vi "Go.vi"(9 "Timing Data":T1(array[cluster]), 10 "Control In":T2={"I-O.lvclass"=refnum, "Gantry"=refnum, "Dispenser"="COM1"}, 11 "Sensor Dispense in":refnum<class "Sensor Dispense.lvclass">) -> (2 "Control Out":T2={"I-O.lvclass"=refnum, "Gantry"=refnum, "Dispenser"="COM1"}, 3 "Sensor Dispense out":refnum<class "Sensor Dispense.lvclass">)   [LabVIEW 2021, in "Sensor Dispense.lvclass"]
uses:
  Sensor Dispense.lvclass
  C:/Users/HEP/Documents/GitHub/Gantry/UCSB-Gantry-HEP-main/Classes/Routine/Dispense/Dispense.lvclass
  Classes/Controller/Controllers.ctl
  Classes/Controller/I-O/I-O.lvclass
  C:/Program Files (x86)/Aerotech/A3200/LabVIEW/2010/Bin/Aerotech.A3200.dll
  Program Files (x86)/Aerotech/A3200/LabVIEW/2010/Bin/Aerotech.A3200.dll
  Sensor Dispense.lvclass/Sensor Dispense.ctl
  Classes/Controller/Motion/Motion.lvclass
  Classes/Controller/Dispenser/Dispenser.lvclass
  Classes/Controller/Motion/A3200/A3200.lvclass
  Classes/Controller/Controller.lvclass
panel:
  out "error out":errorcluster
  in  "error in (no error)":errorcluster
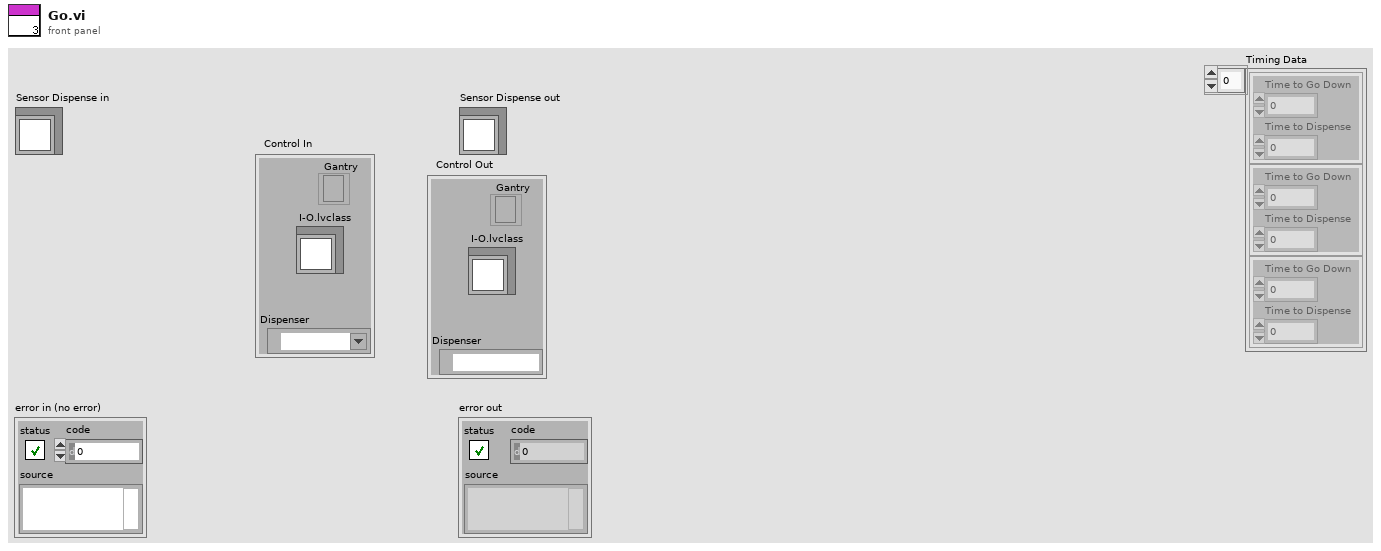
[diagram p1: front panel]
types:
  T1 = cluster{"Time to Go Down":i32, "Time to Dispense":i32}[]
  T2 = typedef "Controller.lvclass/Controllers.ctl" = cluster{"I-O.lvclass":refnum<class "I-O.lvclass">, "Gantry":refnum<k24>, "Dispenser":refnum<visa-resource-name>}
  T3 = cluster{"Endpoints":dbl[][], "Center":dbl[], "CW/CCW":dbl, "Dispense Type":enum16{"N-gon", "Square", "Arc", "Dot", "Line", "Circle"}}[]
  T4 = cluster{"Endpoints":dbl[][], "Center":dbl[], "CW/CCW":dbl, "Dispense Type":enum16{"N-gon", "Square", "Arc", "Dot", "Line", "Circle"}}
  T5 = enum16{"N-gon", "Square", "Arc", "Dot", "Line", "Circle"}
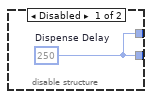
[diagram p2: hidden frame]
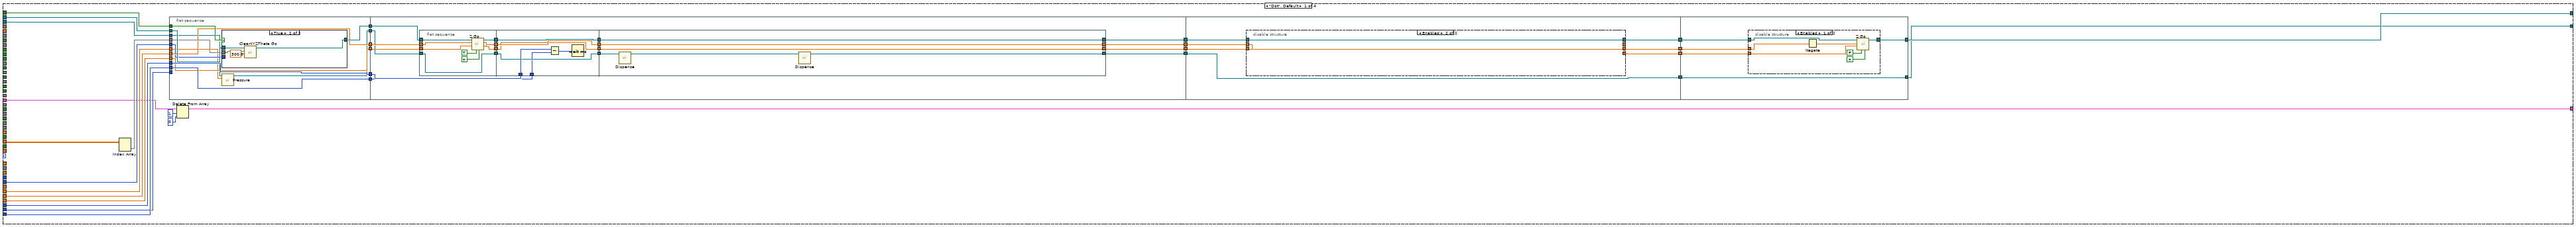
[diagram p4: hidden frame]
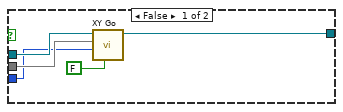
[diagram p5: hidden frame]
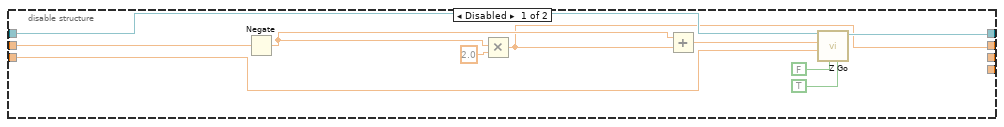
[diagram p6: hidden frame]
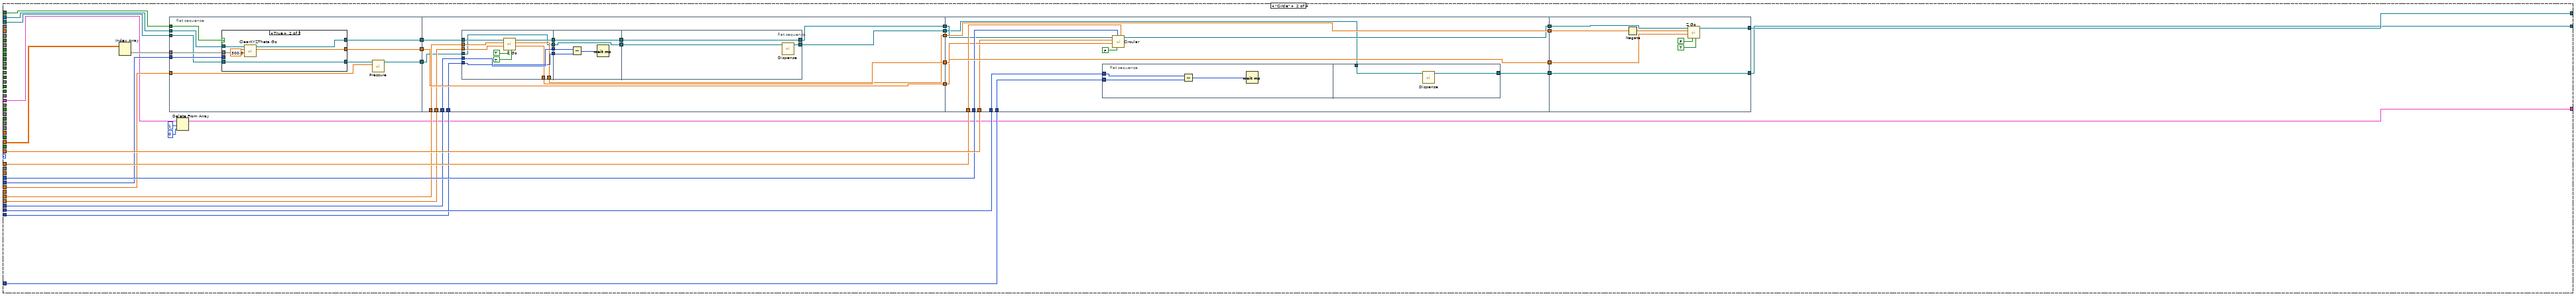
[diagram p8: hidden frame]
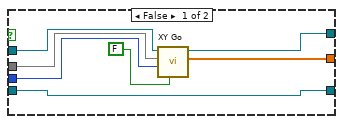
[diagram p9: hidden frame]
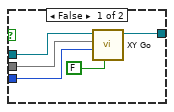
[diagram p10: hidden frame]
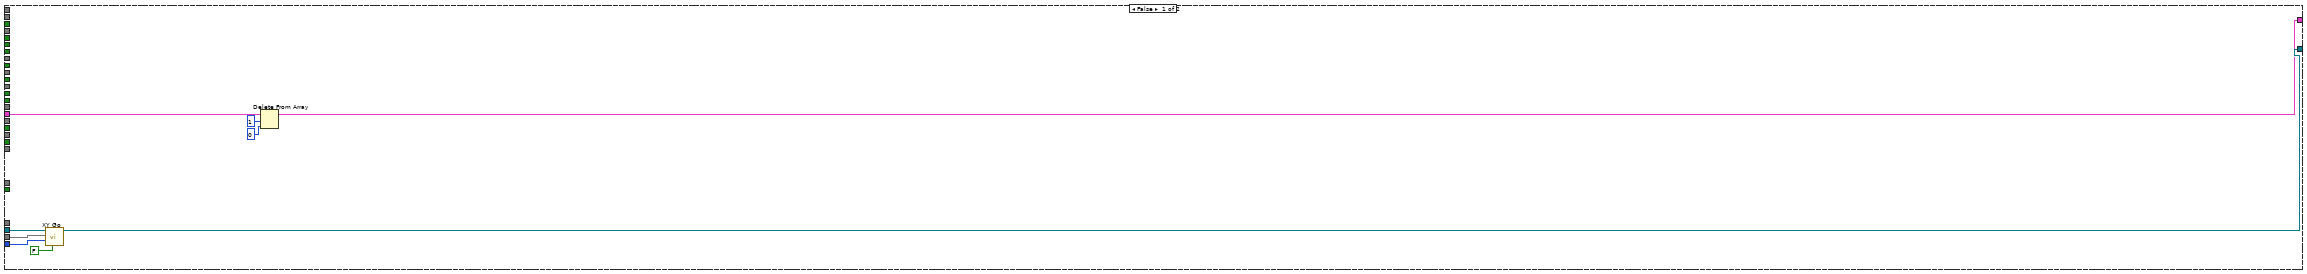
[diagram p11: hidden frame]
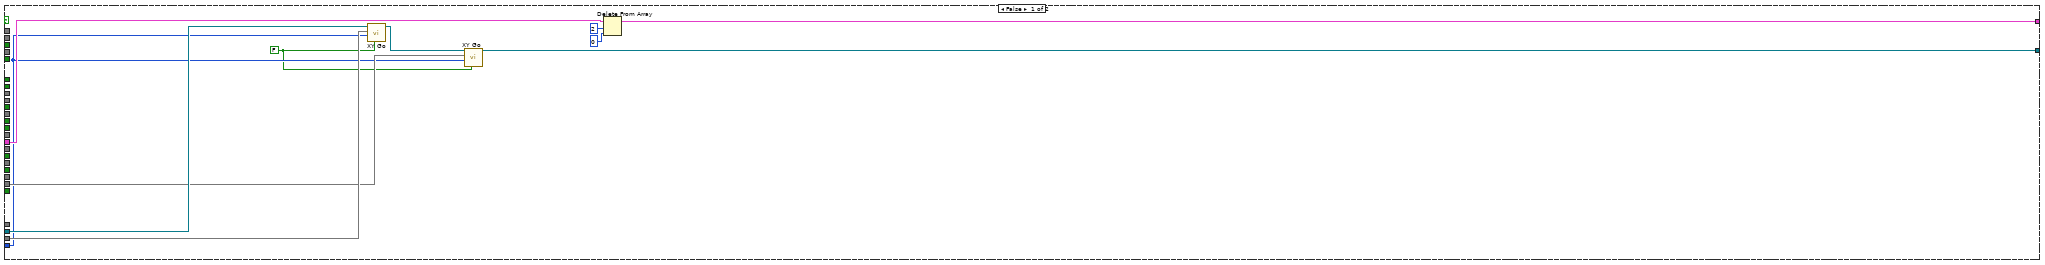
[diagram p12: hidden frame]
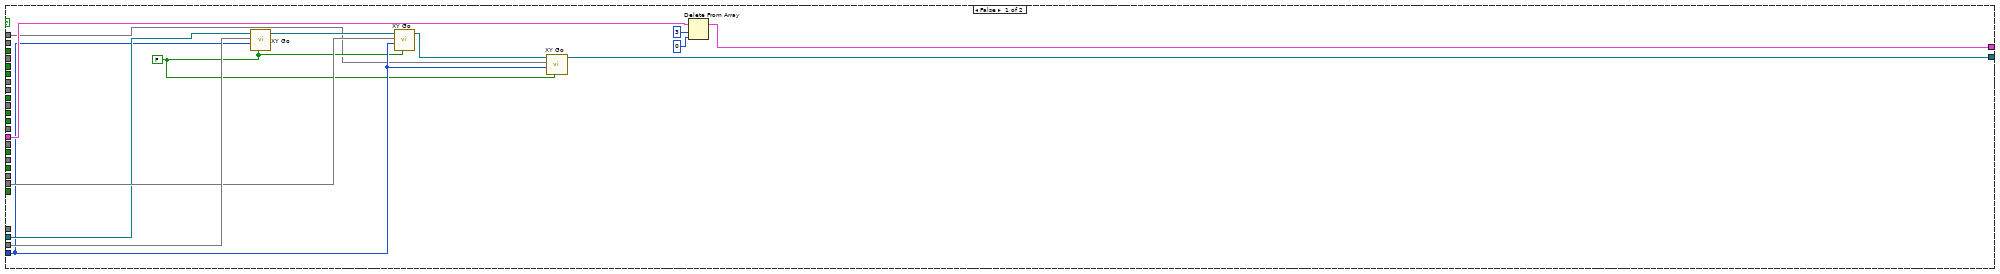
[diagram p13: hidden frame]
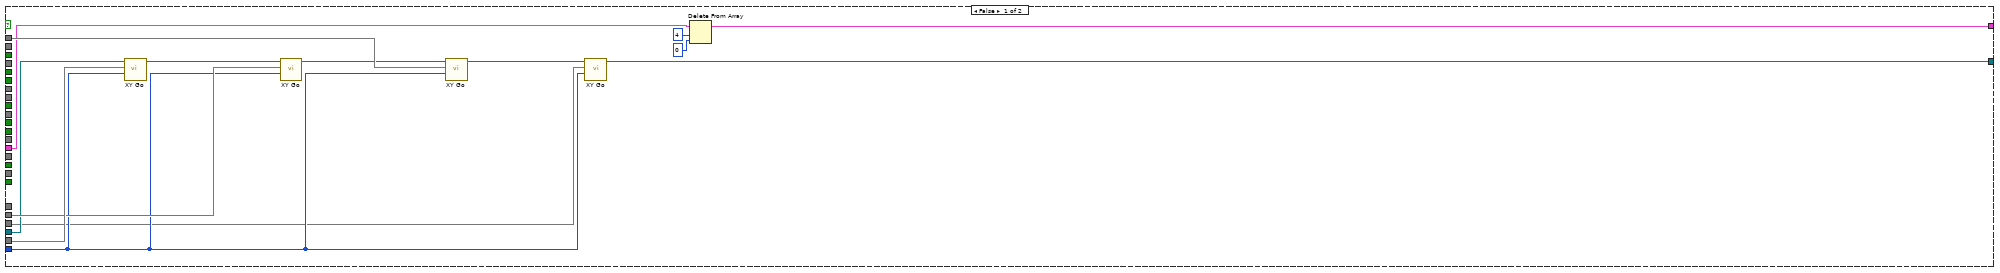
[diagram p14: hidden frame]
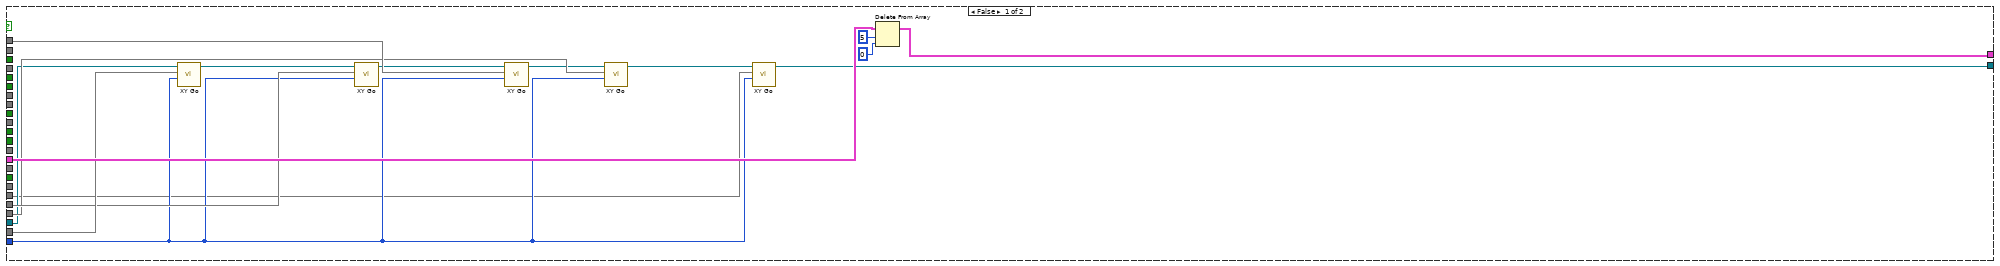
[diagram p15: hidden frame]
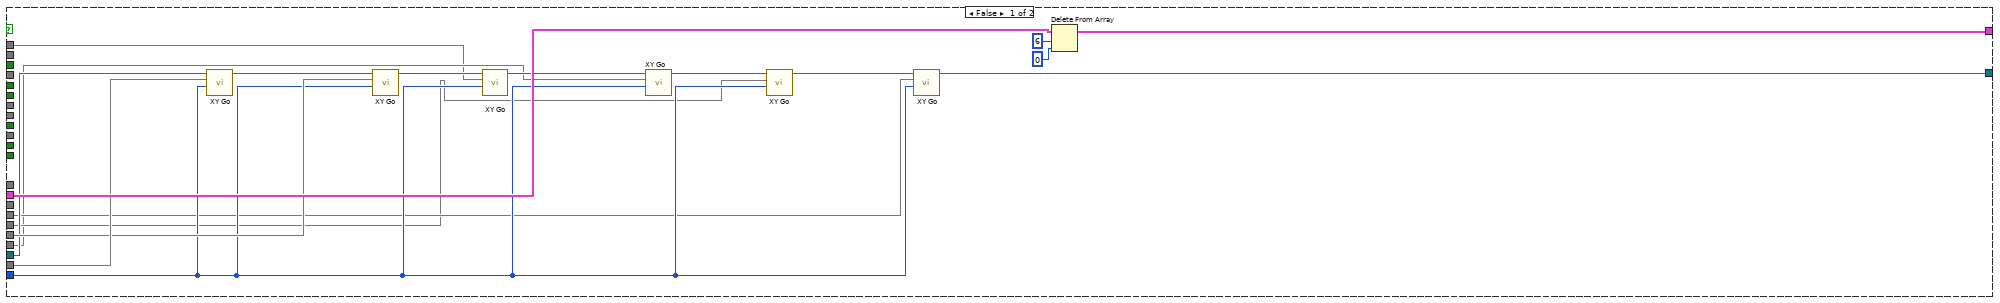
[diagram p16: hidden frame]
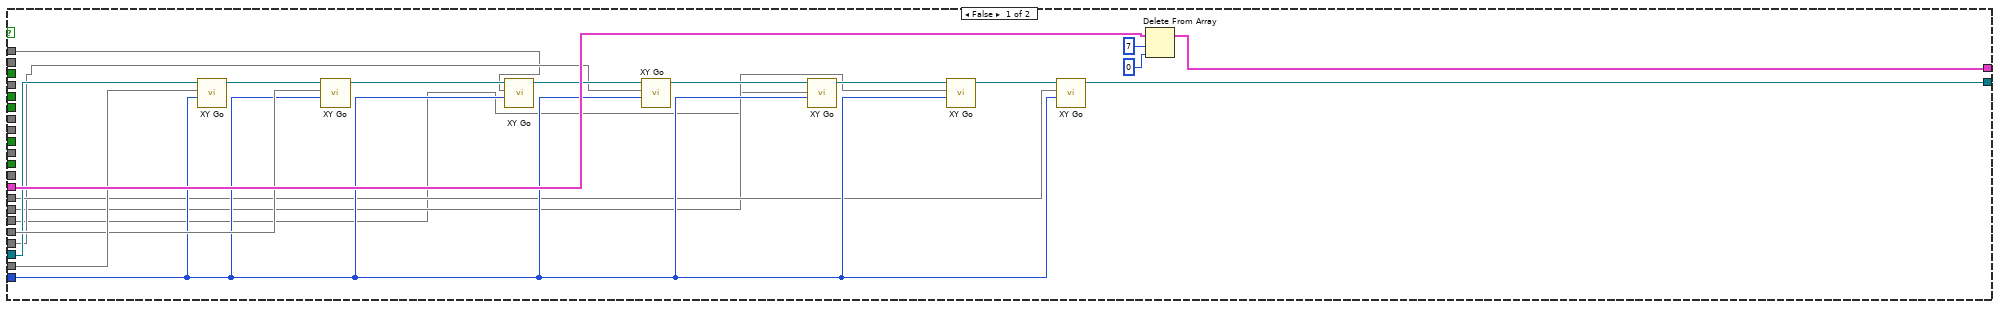
[diagram p17: hidden frame]
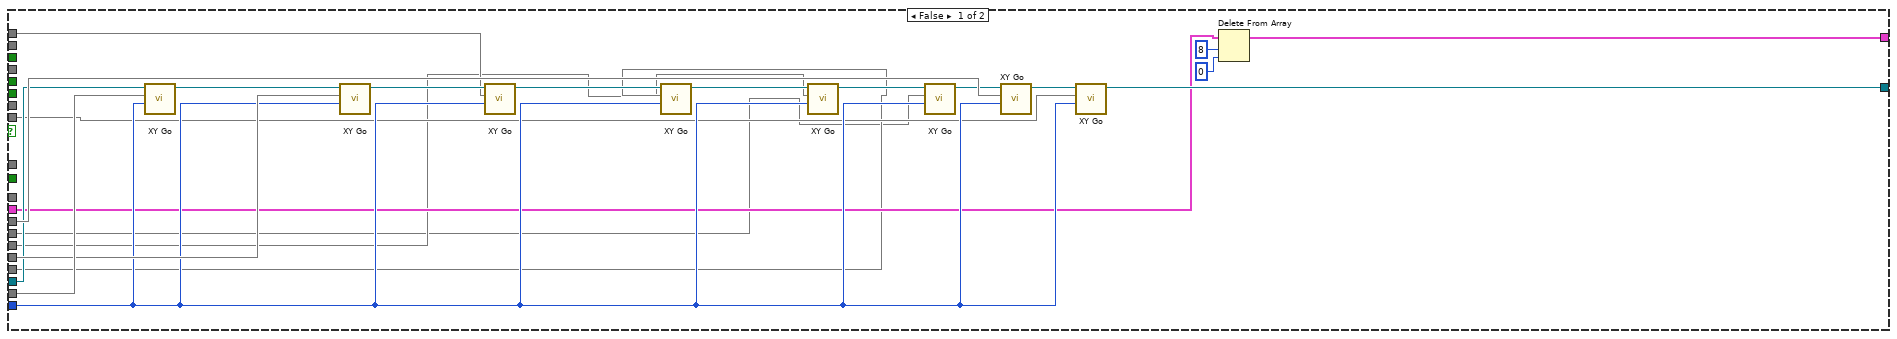
[diagram p18: hidden frame]
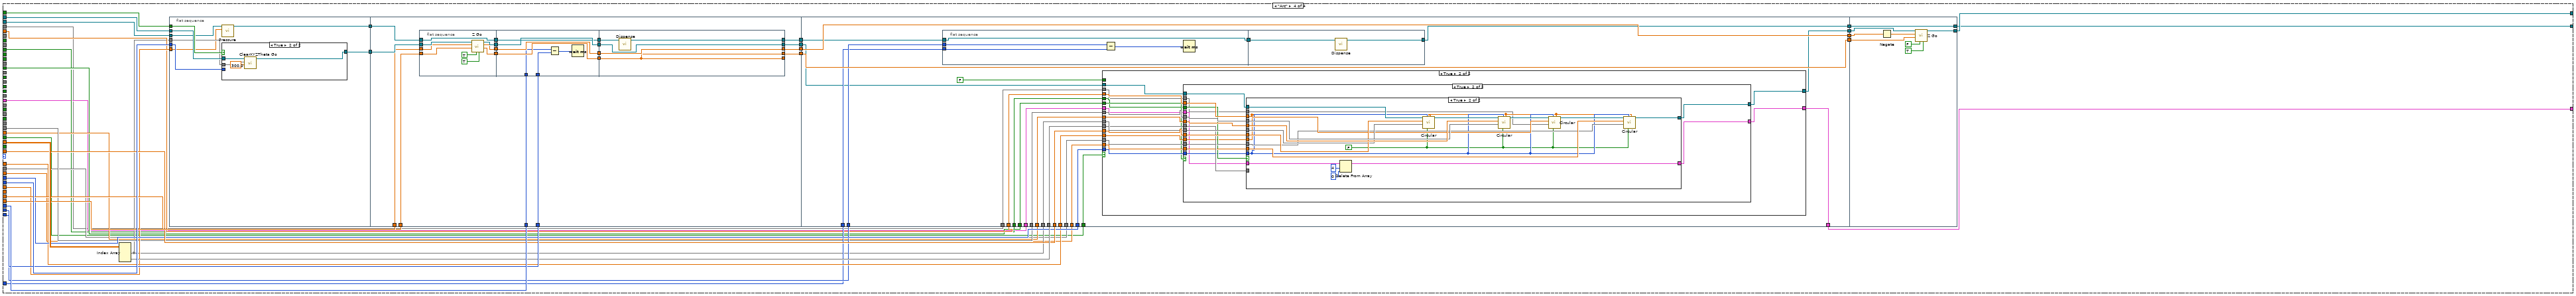
[diagram p19: hidden frame]
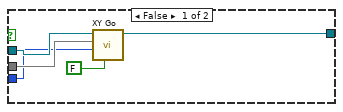
[diagram p20: hidden frame]
diagram:
  n1 = case shown="No Error" "error in (no error)" {
    selector: "error in (no error)" -> [w7 w1398]
    tunnel: "Sensor Dispense in" -> [w12 w1397]
    tunnel: [w11 w1397] -> w5
    tunnel: "Control In" -> [w10 w1396]
    tunnel: [w9 w1396] -> w3
    tunnel: [w8 w1398] -> w2
    frame No Error {
      n2 = in-place {
        in-place-border: w12 -> [w24]
        in-place-border: [w23] -> w11
        in-place-border: w7 -> [w17]
        in-place-border: [w16] -> w8
        n3 = in-place-cluster #1(w10) -> ("Gantry"=w25:refnum<k24>, "Dispenser"=w20:refnum<visa-resource-name>)
        n4 = Unbundle By Name(w24) -> ("Dispense Steps"=w21:T3, "Glue Speed"=w15:i32, "Move Speed"=w26:i32, "Line Pressure"=w13:dbl, "Dot Pressure"=w14:dbl)
        n5 = while {
          tunnel: w26 -> [w170]
          shift-right: [w163] -> w22
          shift-left: w25 -> [w31]
          tunnel: w15 -> [w169]
          shift-right: [w155] -> w23
          shift-left: w24 -> [w167]
          shift-right: [w158] -> w18
          shift-left: w20 -> [w161]
          tunnel: "Timing Data" -> [w160] mode=indexing
          shift-right: [w29] -> w16
          shift-left: w17 -> [w28]
          tunnel: w14 -> [w153]
          tunnel: w13 -> [w152]
          shift-right: [w116] -> _
          shift-left: w21 -> [w68]
          i -> [w166]
          stop <- w118 stop-if-true
          # "740 is good"
          # "compares 3 and 4"
          # "compares 2 and 3"
          # "Compares 1 and 2"
          # "#2"
          # "#3"
          # "#4"
          # "#3"
          # "1/11/23 - Originally 750"
          n6 = Unbundle By Name(w160) -> ("Time to Go Down"=w159:i32, "Time to Dispense"=w150:i32)
          n7 = call "get Estop status.vi"("error in (no error)"=w28, "controller in"=w31) -> ("error out"=w29:errorcluster, "Estop?"=w27:bool, "controller out"=w30:refnum<k24>)  [unwired: 7 in]
          n8 = disable-structure shown="Enabled" {
            disable-tunnel: [w171 w175] -> w154
            disable-tunnel: [w171 w173] -> w151
            disable-tunnel: w150 -> [_ w174]
            frame Disabled {
              w171 = 250  # Dispense Delay
            }
            frame Enabled {
              w172 = 450  # End Dispense Delay
              w175 = 740  # Start Dispense Delay
              # "For arcs it is set to 250"
              # "525 - 1/23/2023"
              # "Originally 0"
              n9 = disable-structure shown="Disabled" {
                disable-tunnel: w174 -> [w180 _]
                disable-tunnel: [w177 w181] -> w173
                disable-tunnel: w172 -> [w176 w181]
                frame Disabled {
                  n10 = Less?(x=w180, y=w176) -> (x < y?=w179:bool)
                  n11 = Select(t=0, s=w179, f=w176) -> (s? t:f=w177:i32)
                }
                frame Enabled {
                }
              }
            }
          }
          n12 = Stop(stop? (T)=w27) -> ()
          n13 = Index Array(array=w68) -> (element=w148:T4)  [unwired: 1 in]
          n14 = Index Array(array=w68, index=11) -> (element=w74:T4)
          n15 = Index Array(array=w68, index=7) -> (element=w109:T4)
          n16 = Index Array(array=w68, index=9) -> (element=w80:T4)
          n17 = Index Array(array=w68, index=10) -> (element=w77:T4)
          n18 = Index Array(array=w68, index=12) -> (element=w71:T4)
          n19 = Index Array(array=w68, index=2) -> (element=w145:T4)
          n20 = Index Array(array=w68, index=8) -> (element=w83:T4)
          n21 = Index Array(array=w68, index=4) -> (element=w115:T4)
          n22 = Index Array(array=w68, index=6) -> (element=w111:T4)
          n23 = Index Array(array=w68, index=5) -> (element=w113:T4)
          n24 = Index Array(array=w68, index=1) -> (element=w147:T4)
          n25 = Index Array(array=w68, index=3) -> (element=w144:T4)
          n26 = Unbundle By Name(w145) -> ("Endpoints"=w142:dbl[][], "Center"=w123:dbl[])
          n27 = Unbundle By Name(w80) -> ("Endpoints"=w79:dbl[][])  [unwired: 1 out]
          n28 = Unbundle By Name(w109) -> ("Endpoints"=w108:dbl[][])  [unwired: 1 out]
          n29 = Unbundle By Name(w83) -> ("Endpoints"=w82:dbl[][])  [unwired: 1 out]
          n30 = Unbundle By Name(w115) -> ("Endpoints"=w114:dbl[][])  [unwired: 1 out]
          n31 = Unbundle By Name(w148) -> ("Endpoints"=w139:dbl[][], "Center"=w162:dbl[], "Dispense Type"=w164:T5, "CW/CCW"=w168:dbl)
          n32 = Unbundle By Name(w111) -> ("Endpoints"=w110:dbl[][])  [unwired: 1 out]
          n33 = Unbundle By Name(w144) -> ("Endpoints"=w143:dbl[][], "Center"=w122:dbl[])
          n34 = Unbundle By Name(w113) -> ("Endpoints"=w112:dbl[][])  [unwired: 1 out]
          n35 = Unbundle By Name(w147) -> ("Endpoints"=w146:dbl[][], "Center"=w124:dbl[])
          n36 = Unbundle By Name(w74) -> ("Endpoints"=w73:dbl[][])  [unwired: 1 out]
          n37 = Unbundle By Name(w77) -> ("Endpoints"=w76:dbl[][])  [unwired: 1 out]
          n38 = Unbundle By Name(w71) -> ("Endpoints"=w70:dbl[][])  [unwired: 1 out]
          n39 = Index Array(array=w108) -> (element #1=w87:dbl[], element #2=w66:dbl[])  [unwired: 4 in]
          n40 = Index Array(array=w142) -> (element #1=w136:dbl[], element #2=w32:dbl[])  [unwired: 4 in]
          n41 = Index Array(array=w112) -> (element #1=w98:dbl[], element #2=w36:dbl[])  [unwired: 4 in]
          n42 = Index Array(array=w143) -> (element #1=w135:dbl[], element #2=w33:dbl[])  [unwired: 4 in]
          n43 = Index Array(array=w82) -> (element #1=w67:dbl[], element #2=w60:dbl[])  [unwired: 4 in]
          n44 = Index Array(array=w79) -> (element #1=w61:dbl[], element #2=w54:dbl[])  [unwired: 4 in]
          n45 = Index Array(array=w114) -> (element #1=w103:dbl[], element #2=w35:dbl[])  [unwired: 4 in]
          n46 = Index Array(array=w110) -> (element #1=w93:dbl[], element #2=w34:dbl[])  [unwired: 4 in]
          n47 = Index Array(array=w146) -> (element #1=w137:dbl[], element #2=w125:dbl[])  [unwired: 4 in]
          n48 = Index Array(array=w73) -> (element #1=w48:dbl[], element #2=w43:dbl[])  [unwired: 4 in]
          n49 = Index Array(array=w76) -> (element #1=w55:dbl[], element #2=w49:dbl[])  [unwired: 4 in]
          n50 = Index Array(array=w70) -> (element #1=w42:dbl[], element #2=w37:dbl[])  [unwired: 4 in]
          n51 = Index Array(array=w139) -> (element #2=w138:dbl[])  [unwired: 4 in, 1 out]
          n52 = Equal?(x=w43, y=w42) -> (x = y?=w41:bool[])
          n53 = Equal?(x=w49, y=w48) -> (x = y?=w47:bool[])
          n54 = Equal?(x=w54, y=w55) -> (x = y?=w53:bool[])
          n55 = Equal?(x=w125, y=w136) -> (x = y?=w131:bool[])
          n56 = Equal?(x=w66, y=w67) -> (x = y?=w65:bool[])
          n57 = Equal?(x=w60, y=w61) -> (x = y?=w59:bool[])
          n58 = Equal?(x=w34, y=w87) -> (x = y?=w88:bool[])
          n59 = Equal?(x=w36, y=w93) -> (x = y?=w92:bool[])
          n60 = Equal?(x=w35, y=w98) -> (x = y?=w97:bool[])
          n61 = Equal?(x=w33, y=w103) -> (x = y?=w102:bool[])
          n62 = Equal?(x=w32, y=w135) -> (x = y?=w130:bool[])
          n63 = Index Array(array=w130) -> (element #1=w127:bool, element #2=w126:bool)  [unwired: 2 in]
          n64 = And(x=w127, y=w126) -> (x .and. y?=w119:bool)
          n65 = Index Array(array=w41) -> (element #1=w40:bool, element #2=w39:bool)  [unwired: 2 in]
          n66 = Equal?(x=w138, y=w137) -> (x = y?=w134:bool[])
          n67 = Index Array(array=w53) -> (element #1=w52:bool, element #2=w51:bool)  [unwired: 2 in]
          n68 = Index Array(array=w131) -> (element #1=w129:bool, element #2=w128:bool)  [unwired: 2 in]
          n69 = Index Array(array=w65) -> (element #1=w64:bool, element #2=w63:bool)  [unwired: 2 in]
          n70 = Index Array(array=w59) -> (element #1=w58:bool, element #2=w57:bool)  [unwired: 2 in]
          n71 = Index Array(array=w88) -> (element #1=w86:bool, element #2=w85:bool)  [unwired: 2 in]
          n72 = Index Array(array=w92) -> (element #1=w91:bool, element #2=w90:bool)  [unwired: 2 in]
          n73 = Index Array(array=w97) -> (element #1=w96:bool, element #2=w95:bool)  [unwired: 2 in]
          n74 = property on="Property Node" class="Sensor Dispense.lvclass"(reference=w167) -> (reference out=w155:refnum<class "Sensor Dispense.lvclass">, "Z height"=w157:dbl, "Z speed"=w156:dbl)  [unwired: 1 in, 1 out]
          n75 = Index Array(array=w47) -> (element #1=w46:bool, element #2=w45:bool)  [unwired: 2 in]
          n76 = Index Array(array=w102) -> (element #1=w101:bool, element #2=w100:bool)  [unwired: 2 in]
          n77 = And(x=w40, y=w39) -> (x .and. y?=w38:bool)
          n78 = Index Array(array=w134) -> (element #1=w133:bool, element #2=w132:bool)  [unwired: 2 in]
          n79 = And(x=w46, y=w45) -> (x .and. y?=w44:bool)
          n80 = And(x=w52, y=w51) -> (x .and. y?=w50:bool)
          n81 = And(x=w64, y=w63) -> (x .and. y?=w62:bool)
          n82 = And(x=w58, y=w57) -> (x .and. y?=w56:bool)
          n83 = And(x=w86, y=w85) -> (x .and. y?=w84:bool)
          n84 = And(x=w91, y=w90) -> (x .and. y?=w89:bool)
          n85 = And(x=w96, y=w95) -> (x .and. y?=w94:bool)
          n86 = And(x=w101, y=w100) -> (x .and. y?=w99:bool)
          n87 = And(x=w129, y=w128) -> (x .and. y?=w120:bool)
          n88 = And(x=w133, y=w132) -> (x .and. y?=w121:bool)
          n89 = Equal To 0?(x=w166) -> (x = 0?=w165:bool)
          n90 = case shown="\"Line\"" w164 {
            tunnel: w162 -> [_ w337 _ w1187]
            tunnel: w30 -> [w212 w338 w489 w1195]
            tunnel: w170 -> [w195 w331 w488 w1193]
            tunnel: [w211 w341 w485 w1183] -> w163
            tunnel: w169 -> [_ w336 w476 w1186]
            tunnel: w168 -> [_ w335 _ w1185]
            tunnel: w156 -> [w203 w333 w473 w1189]
            tunnel: w157 -> [w204 w334 w474 w1190]
            tunnel: w165 -> [w213 w332 w487 w1196]
            tunnel: w161 -> [w202 w315 w480 w1179]
            tunnel: w159 -> [w200 w322 w478 w1192]
            tunnel: w150 -> [w205 w323 w475 w1184]
            tunnel: w154 -> [w206 w321 w479 w1191]
            tunnel: [w210 w316 w483 w1182] -> w158
            tunnel: w139 -> [w209 w320 w482 w1194]
            tunnel: w153 -> [w194 _ _ _]
            tunnel: w152 -> [_ w313 w456 w1178]
            tunnel: w151 -> [_ w312 w455 w1177]
            tunnel: w125 -> [_ _ w452 w1176]
            tunnel: w124 -> [_ _ _ w1175]
            tunnel: w123 -> [_ _ _ w1174]
            tunnel: w122 -> [_ _ _ w1172]
            tunnel: w33 -> [_ _ w447 w1171]
            tunnel: w121 -> [_ _ w450 w1170]
            tunnel: w120 -> [_ _ w449 w1169]
            tunnel: w119 -> [_ _ w448 w1168]
            tunnel: w68 -> [w186 w311 w453 w1167]
            tunnel: [w183 w308 w454 w1166] -> w116
            tunnel: w32 -> [_ _ w451 w1165]
            tunnel: w99 -> [_ _ w446 _]
            tunnel: w35 -> [_ _ w445 _]
            tunnel: w94 -> [_ _ w444 _]
            tunnel: w36 -> [_ _ w443 _]
            tunnel: w89 -> [_ _ w442 _]
            tunnel: w84 -> [_ _ w441 _]
            tunnel: w34 -> [_ _ w440 _]
            tunnel: w66 -> [_ _ w439 _]
            tunnel: w62 -> [_ _ w438 _]
            tunnel: w60 -> [_ _ w437 _]
            tunnel: w56 -> [_ _ w436 _]
            tunnel: w54 -> [_ _ w435 _]
            tunnel: w50 -> [_ _ w434 _]
            tunnel: w49 -> [_ _ w433 _]
            tunnel: w44 -> [_ _ w432 _]
            tunnel: w43 -> [_ _ w431 _]
            tunnel: w38 -> [_ _ w430 _]
            tunnel: w37 -> [_ _ w429 _]
            frame "Dot", Default {
              n91 = Index Array(array=w209) -> (element=w208:dbl[])  [unwired: 2 in]
              n92 = flat-sequence {
                tunnel: w213 -> [w225]
                tunnel: w212 -> [w224]
                tunnel: w208 -> [w223]
                tunnel: [w222] -> w207
                tunnel: w206 -> [w219]
                tunnel: w205 -> [_]
                tunnel: w204 -> [w221]
                tunnel: w203 -> [w218]
                tunnel: w202 -> [w216]
                tunnel: [w221] -> w201
                tunnel: w200 -> [w220]
                tunnel: [w220] -> w199
                tunnel: [w219] -> w198
                tunnel: [w215] -> w197
                tunnel: [w218] -> w196
                tunnel: w195 -> [w217]
                tunnel: w194 -> [w214]
                tunnel: [w252] -> w191
                tunnel: w207 -> [w251]
                tunnel: [w248] -> w190
                tunnel: w201 -> [w247]
                tunnel: w199 -> [w246]
                tunnel: w198 -> [w245]
                tunnel: w197 -> [w244]
                tunnel: w196 -> [w241]
                tunnel: [w239] -> w189
                tunnel: [w238] -> w188
                tunnel: w191 -> [w280]
                tunnel: w190 -> [w279]
                tunnel: w189 -> [w278]
                tunnel: w188 -> [w277]
                tunnel: [w281] -> w193
                tunnel: [w280] -> w192
                tunnel: [w275] -> w187
                tunnel: [w276] -> w182
                tunnel: [w295] -> w210
                tunnel: [w298] -> w211
                tunnel: w193 -> [w299]
                tunnel: w192 -> [w295]
                tunnel: w187 -> [w297]
                tunnel: w182 -> [w296]
                frame #0 {
                  n93 = case shown="True" w225 {
                    tunnel: w224 -> [w230 w234]
                    tunnel: [w229 w233] -> w222
                    tunnel: w223 -> [w228 w232]
                    tunnel: w217 -> [w227 _]
                    frame False {
                      n94 = call "XY Go.vi"("return immediately"=FALSE, "Speed"=w227, "XY In"=w228, "Gantry In"=w230) -> ("Gantry Out"=w229:refnum<k24>)  [unwired: 5 in, 2 out]
                    }
                    frame True {
                      n95 = call "ClearXYZTheta Go.vi"("Speed"=300.0, "XYZTheta In"=w232, "Gantry In"=w234) -> ("Gantry Out"=w233:refnum<k24>)  [unwired: 6 in, 2 out]
                    }
                  }
                  n96 = call "Pressure.vi"("Pressure"=w214, "VISA resource name"=w216) -> ("VISA resource name out"=w215:refnum<visa-resource-name>)  [unwired: 8 in, 1 out]
                }
                frame #1 {
                  n97 = flat-sequence {
                    tunnel: w251 -> [w261]
                    tunnel: [w260] -> w249
                    tunnel: w247 -> [w254]
                    tunnel: w244 -> [w258]
                    tunnel: [w258] -> w243
                    tunnel: w241 -> [w257]
                    tunnel: [w256] -> w236
                    tunnel: [w253] -> w235
                    tunnel: [w268] -> w250
                    tunnel: w249 -> [w268]
                    tunnel: w246 -> [w267]
                    tunnel: w245 -> [w263]
                    tunnel: w243 -> [w266]
                    tunnel: [w266] -> w242
                    tunnel: [w265] -> w240
                    tunnel: [w264] -> w237
                    tunnel: w236 -> [w264]
                    tunnel: w235 -> [w265]
                    tunnel: [w274] -> w252
                    tunnel: w250 -> [w273]
                    tunnel: [w273] -> w248
                    tunnel: w242 -> [w272]
                    tunnel: w240 -> [w270]
                    tunnel: [w270] -> w239
                    tunnel: [w269] -> w238
                    tunnel: w237 -> [w269]
                    frame #0 {
                      n98 = call "Z Go.vi"("Increment"=TRUE, "Return Immediately"=TRUE, "Speed In"=w257, "Position In"=w254, "Gantry In"=w261) -> ("Speed Out"=w256:dbl, "Position Out"=w253:dbl, "Gantry Out"=w260:refnum<k24>)  [unwired: 3 in, 1 out]
                    }
                    frame #1 {
                      n99 = Subtract(x=w267, y=w263) -> (x-y=w262:i32)
                      n100 = Wait (ms)(milliseconds to wait=w262) -> ()  [unwired: 1 out]
                    }
                    frame #2 {
                      n101 = call "Dispense.vi"("Dispenser In"=w272) -> ("Dispenser Out"=w271:refnum<visa-resource-name>)  [unwired: 9 in, 1 out]
                      n102 = call "Dispense.vi"("Dispenser In"=w271) -> ("Dispenser Out"=w274:refnum<visa-resource-name>)  [unwired: 9 in, 1 out]
                    }
                  }
                }
                frame #2 {
                  n103 = disable-structure shown="Enabled" {
                    disable-tunnel: [w291 w294] -> w281
                    disable-tunnel: w279 -> [w290 w294]
                    disable-tunnel: w278 -> [w289 w292]
                    disable-tunnel: w277 -> [w286 w293]
                    disable-tunnel: [w282 _] -> _
                    disable-tunnel: [_ w293] -> w276
                    disable-tunnel: [_ w292] -> w275
                    frame Disabled {
                      n104 = Negate(x=w289) -> (-x=w284:dbl)
                      n105 = Multiply(x=w284, y=2.0) -> (x*y=w282:dbl)
                      n106 = Add(x=w284, y=w282) -> (x+y=w285:dbl)
                      n107 = call "Z Go.vi"("Increment"=TRUE, "Return Immediately"=FALSE, "Speed In"=w286, "Position In"=w285, "Gantry In"=w290) -> ("Gantry Out"=w291:refnum<k24>)  [unwired: 3 in, 3 out]
                    }
                    frame Enabled {
                    }
                  }
                }
                frame #3 {
                  n108 = disable-structure shown="Enabled" {
                    disable-tunnel: w299 -> [w306 w307]
                    disable-tunnel: [w305 w307] -> w298
                    disable-tunnel: w297 -> [w300 _]
                    disable-tunnel: w296 -> [w301 _]
                    frame Enabled {
                      n109 = Negate(x=w300) -> (-x=w304:dbl)
                      n110 = call "Z Go.vi"("Increment"=TRUE, "Return Immediately"=FALSE, "Speed In"=w301, "Position In"=w304, "Gantry In"=w306) -> ("Gantry Out"=w305:refnum<k24>)  [unwired: 3 in, 3 out]
                    }
                    frame Disabled {
                    }
                  }
                }
              }
              n111 = Delete From Array(array=w186, length=1, index=0) -> (array with subset deleted=w183:T3)  [unwired: 1 out]
            }
            frame "Circle" {
              n112 = Index Array(array=w320) -> (element=w319:dbl[])  [unwired: 2 in]
              n113 = flat-sequence {
                tunnel: [w349] -> w340
                tunnel: w338 -> [w350]
                tunnel: w332 -> [w351]
                tunnel: w331 -> [w348]
                tunnel: [w347] -> w329
                tunnel: w319 -> [w346]
                tunnel: w315 -> [w345]
                tunnel: [w343] -> w314
                tunnel: w313 -> [w342]
                tunnel: w334 -> [w374]
                tunnel: w333 -> [w375]
                tunnel: [w381] -> w330
                tunnel: [w372] -> w328
                tunnel: [w373] -> w327
                tunnel: w329 -> [w381]
                tunnel: w340 -> [w371]
                tunnel: [w380] -> w324
                tunnel: w322 -> [w379]
                tunnel: w321 -> [w378]
                tunnel: [w368] -> w318
                tunnel: w314 -> [w367]
                tunnel: [w403] -> w339
                tunnel: [w413] -> w326
                tunnel: [w412] -> w325
                tunnel: w323 -> [w411]
                tunnel: w324 -> [w401]
                tunnel: w330 -> [w406]
                tunnel: w328 -> [w413]
                tunnel: w327 -> [w412]
                tunnel: w335 -> [w409]
                tunnel: w336 -> [w407]
                tunnel: w337 -> [w405]
                tunnel: w318 -> [w404]
                tunnel: [w410] -> w317
                tunnel: w312 -> [w402]
                tunnel: [w424] -> w341
                tunnel: w339 -> [w425]
                tunnel: w326 -> [w426]
                tunnel: w325 -> [w423]
                tunnel: w317 -> [w422]
                tunnel: [w422] -> w316
                frame #0 {
                  n114 = case shown="True" w351 {
                    tunnel: w350 -> [w358 w364]
                    tunnel: [w357 w363] -> w349
                    tunnel: w348 -> [w356 _]
                    tunnel: [w355 w361] -> w347
                    tunnel: w346 -> [w354 w362]
                    tunnel: w345 -> [w353 w360]
                    tunnel: [w353 w360] -> w344
                    frame False {
                      n115 = call "XY Go.vi"("return immediately"=FALSE, "Speed"=w356, "XY In"=w354, "Gantry In"=w358) -> ("XY Out"=w355:dbl[], "Gantry Out"=w357:refnum<k24>)  [unwired: 5 in, 1 out]
                    }
                    frame True {
                      n116 = call "ClearXYZTheta Go.vi"("Speed"=300.0, "XYZTheta In"=w362, "Gantry In"=w364) -> ("XYZTheta Out"=w361:dbl[], "Gantry Out"=w363:refnum<k24>)  [unwired: 6 in, 1 out]
                    }
                  }
                  n117 = call "Pressure.vi"("Pressure"=w342, "VISA resource name"=w344) -> ("VISA resource name out"=w343:refnum<visa-resource-name>)  [unwired: 8 in, 1 out]
                }
                frame #1 {
                  n118 = flat-sequence {
                    tunnel: w378 -> [w391]
                    tunnel: w379 -> [w392]
                    tunnel: [w392] -> w377
                    tunnel: [w391] -> w376
                    tunnel: w375 -> [w390]
                    tunnel: w374 -> [w389]
                    tunnel: [w388] -> w373
                    tunnel: [w387] -> w372
                    tunnel: w371 -> [w386]
                    tunnel: [w385] -> w370
                    tunnel: w367 -> [w383]
                    tunnel: [w383] -> w366
                    tunnel: w377 -> [w397]
                    tunnel: w376 -> [w396]
                    tunnel: w370 -> [w395]
                    tunnel: [w395] -> w369
                    tunnel: w366 -> [w394]
                    tunnel: [w394] -> w365
                    tunnel: [w400] -> w380
                    tunnel: w369 -> [w399]
                    tunnel: [w399] -> w368
                    tunnel: w365 -> [w398]
                    frame #0 {
                      n119 = call "Z Go.vi"("Increment"=TRUE, "Return Immediately"=TRUE ("return immediately"), "Speed In"=w390, "Position In"=w389, "Gantry In"=w386) -> ("Speed Out"=w388:dbl, "Position Out"=w387:dbl, "Gantry Out"=w385:refnum<k24>)  [unwired: 3 in, 1 out]
                    }
                    frame #1 {
                      n120 = Subtract(x=w397, y=w396) -> (x-y=w393:i32)
                      n121 = Wait (ms)(milliseconds to wait=w393) -> ()  [unwired: 1 out]
                    }
                    frame #2 {
                      n122 = call "Dispense.vi"("Dispenser In"=w398) -> ("Dispenser Out"=w400:refnum<visa-resource-name>)  [unwired: 9 in, 1 out]
                    }
                  }
                }
                frame #2 {
                  n123 = flat-sequence {
                    tunnel: w411 -> [w416]
                    tunnel: w402 -> [w414]
                    tunnel: [w418] -> w410
                    tunnel: w401 -> [w417]
                    frame #0 {
                      n124 = Subtract(x=w416, y=w414) -> (x-y=w415:i32)
                      n125 = Wait (ms)(milliseconds to wait=w415) -> ()  [unwired: 1 out]
                    }
                    frame #1 {
                      n126 = call "Dispense.vi"("Dispenser In"=w417) -> ("Dispenser Out"=w418:refnum<visa-resource-name>)  [unwired: 9 in, 1 out]
                    }
                  }
                  n127 = call "Circular.vi"("Direction"=w409, "return immediately"=FALSE, "Speed"=w407, "XY End"=w406, "XY Center"=w405, "Gantry In"=w404) -> ("Gantry Out"=w403:refnum<k24>)  [unwired: 4 in, 1 out]
                }
                frame #3 {
                  n128 = Negate(x=w426) -> (-x=w421:dbl)
                  n129 = call "Z Go.vi"("Increment"=TRUE, "Return Immediately"=FALSE, "Speed In"=w423, "Position In"=w421, "Gantry In"=w425) -> ("Gantry Out"=w424:refnum<k24>)  [unwired: 3 in, 3 out]
                }
              }
              n130 = Delete From Array(array=w311, length=1, index=0) -> (array with subset deleted=w308:T3)  [unwired: 1 out]
            }
            frame "Line" {
              n131 = Index Array(array=w482) -> (element #1=w481:dbl[], element #2=w477:dbl[])  [unwired: 4 in]
              n132 = flat-sequence {
                tunnel: w489 -> [w504]
                tunnel: w488 -> [w503]
                tunnel: w487 -> [w502]
                tunnel: [w501] -> w486
                tunnel: w481 -> [w500]
                tunnel: w480 -> [w492]
                tunnel: w479 -> [w496]
                tunnel: w478 -> [w497]
                tunnel: w477 -> [w495]
                tunnel: w476 -> [w494]
                tunnel: w475 -> [w493]
                tunnel: w474 -> [w499]
                tunnel: w473 -> [w498]
                tunnel: [w499] -> w472
                tunnel: [w498] -> w471
                tunnel: [w497] -> w469
                tunnel: [w496] -> w468
                tunnel: [w491] -> w467
                tunnel: [w495] -> w465
                tunnel: [w494] -> w463
                tunnel: [w493] -> w461
                tunnel: w456 -> [w490]
                tunnel: w486 -> [w537]
                tunnel: w472 -> [w536]
                tunnel: w471 -> [w535]
                tunnel: [w532] -> w470
                tunnel: w469 -> [w529]
                tunnel: w468 -> [w530]
                tunnel: w467 -> [w531]
                tunnel: [w543] -> w466
                tunnel: w465 -> [w542]
                tunnel: [w541] -> w464
                tunnel: w463 -> [w540]
                tunnel: [w538] -> w462
                tunnel: w461 -> [w539]
                tunnel: [w534] -> w458
                tunnel: [w533] -> w428
                tunnel: [w514] -> w427
                tunnel: [w617] -> w484
                tunnel: w470 -> [w606]
                tunnel: w466 -> [w607]
                tunnel: w464 -> [w608]
                tunnel: w462 -> [w615]
                tunnel: [w605] -> w460
                tunnel: [w614] -> w459
                tunnel: w458 -> [w612]
                tunnel: [w611] -> w457
                tunnel: w455 -> [w604]
                tunnel: [w603] -> w454
                tunnel: w453 -> [w602]
                tunnel: w452 -> [w601]
                tunnel: w451 -> [w600]
                tunnel: w450 -> [w599]
                tunnel: w449 -> [w598]
                tunnel: w448 -> [w597]
                tunnel: w447 -> [w596]
                tunnel: w446 -> [w595]
                tunnel: w445 -> [w594]
                tunnel: w444 -> [w593]
                tunnel: w443 -> [w592]
                tunnel: w442 -> [w591]
                tunnel: w441 -> [w590]
                tunnel: w440 -> [w589]
                tunnel: w439 -> [w588]
                tunnel: w438 -> [w587]
                tunnel: w437 -> [w586]
                tunnel: w436 -> [w585]
                tunnel: w435 -> [w584]
                tunnel: w434 -> [w583]
                tunnel: w433 -> [w582]
                tunnel: w432 -> [w581]
                tunnel: w431 -> [w580]
                tunnel: w430 -> [w579]
                tunnel: w429 -> [w578]
                tunnel: w428 -> [w609]
                tunnel: w427 -> [w577]
                tunnel: [w1164] -> w485
                tunnel: w484 -> [w1163]
                tunnel: [w1163] -> w483
                tunnel: w460 -> [w1162]
                tunnel: w459 -> [w1161]
                tunnel: w457 -> [w1159]
                frame #0 {
                  n133 = case shown="True" w502 {
                    tunnel: w504 -> [w509 w513]
                    tunnel: w503 -> [w508 _]
                    tunnel: [w507 w512] -> w501
                    tunnel: w500 -> [w506 w511]
                    frame False {
                      n134 = call "XY Go.vi"("return immediately"=FALSE, "Speed"=w508, "XY In"=w506, "Gantry In"=w509) -> ("Gantry Out"=w507:refnum<k24>)  [unwired: 5 in, 2 out]
                    }
                    frame True {
                      n135 = call "ClearXYZTheta Go.vi"("Speed"=300.0, "XYZTheta In"=w511, "Gantry In"=w513) -> ("Gantry Out"=w512:refnum<k24>)  [unwired: 6 in, 2 out]
                    }
                  }
                  n136 = call "Pressure.vi"("Pressure"=w490, "VISA resource name"=w492) -> ("VISA resource name out"=w491:refnum<visa-resource-name>)  [unwired: 8 in, 1 out]
                }
                frame #1 {
                  n137 = flat-sequence {
                    tunnel: w529 -> [w552]
                    tunnel: w530 -> [w544]
                    tunnel: w542 -> [w551]
                    tunnel: w540 -> [w550]
                    tunnel: w539 -> [w549]
                    tunnel: w537 -> [w560]
                    tunnel: w536 -> [w559]
                    tunnel: w535 -> [w558]
                    tunnel: w531 -> [w546]
                    tunnel: [w552] -> w528
                    tunnel: [w544] -> w527
                    tunnel: [w551] -> w526
                    tunnel: [w550] -> w525
                    tunnel: [w549] -> w524
                    tunnel: [w555] -> w523
                    tunnel: [w554] -> w522
                    tunnel: [w553] -> w521
                    tunnel: [w547] -> w514
                    tunnel: w528 -> [_]
                    tunnel: w527 -> [_]
                    tunnel: w526 -> [w570]
                    tunnel: w525 -> [w569]
                    tunnel: w524 -> [w568]
                    tunnel: w523 -> [w567]
                    tunnel: w522 -> [w566]
                    tunnel: w521 -> [w565]
                    tunnel: [w570] -> w520
                    tunnel: [w569] -> w519
                    tunnel: [w568] -> w518
                    tunnel: [w567] -> w517
                    tunnel: [w566] -> w516
                    tunnel: [w565] -> w515
                    tunnel: [w576] -> w543
                    tunnel: [w575] -> w541
                    tunnel: [w574] -> w538
                    tunnel: [w573] -> w534
                    tunnel: [w572] -> w533
                    tunnel: [w571] -> w532
                    tunnel: w520 -> [w576]
                    tunnel: w519 -> [w575]
                    tunnel: w518 -> [w574]
                    tunnel: w517 -> [w573]
                    tunnel: w516 -> [w572]
                    tunnel: w515 -> [w571]
                    frame #0 {
                      n138 = call "Z Go.vi"("Increment"=TRUE ("Return Immediately"), "Return Immediately"=FALSE ("Increment"), "Speed In"=w558, "Position In"=w559, "Gantry In"=w560) -> ("Speed Out"=w554:dbl, "Position Out"=w555:dbl, "Gantry Out"=w553:refnum<k24>)  [unwired: 3 in, 1 out]
                      n139 = Subtract(x=w552, y=w544) -> (x-y=w548:i32)
                      n140 = flat-sequence {
                        tunnel: w548 -> [w562]
                        tunnel: w546 -> [w561]
                        tunnel: [w561] -> w545
                        tunnel: [w564] -> w547
                        tunnel: w545 -> [w563]
                        frame #0 {
                          n141 = Wait (ms)(milliseconds to wait=w562) -> ()  [unwired: 1 out]
                        }
                        frame #1 {
                          n142 = call "Dispense.vi"("Dispenser In"=w563) -> ("Dispenser Out"=w564:refnum<visa-resource-name>)  [unwired: 9 in, 1 out]
                        }
                      }
                    }
                    frame #1 {
                    }
                    frame #2 {
                    }
                  }
                }
                frame #2 {
                  n143 = case shown="True" w599 {
                    tunnel: w608 -> [w626 w651]
                    tunnel: w607 -> [w625 w654]
                    tunnel: w606 -> [w624 w653]
                    tunnel: [w623 w650] -> w605
                    tunnel: [w620 w649] -> w603
                    tunnel: w602 -> [w621 w655]
                    tunnel: w601 -> [_ w652]
                    tunnel: w600 -> [_ w648]
                    tunnel: w598 -> [_ w647]
                    tunnel: w597 -> [_ w646]
                    tunnel: w596 -> [_ w645]
                    tunnel: w595 -> [_ w644]
                    tunnel: w594 -> [_ w643]
                    tunnel: w593 -> [_ w642]
                    tunnel: w592 -> [_ w641]
                    tunnel: w591 -> [_ w640]
                    tunnel: w590 -> [_ w639]
                    tunnel: w589 -> [_ w638]
                    tunnel: w588 -> [_ w637]
                    tunnel: w587 -> [_ w636]
                    tunnel: w586 -> [_ w635]
                    tunnel: w585 -> [_ w634]
                    tunnel: w584 -> [_ w633]
                    tunnel: w583 -> [_ w632]
                    tunnel: w582 -> [_ w631]
                    tunnel: w581 -> [_ w630]
                    tunnel: w580 -> [_ w629]
                    tunnel: w579 -> [_ w628]
                    tunnel: w578 -> [_ w627]
                    frame False {
                      n144 = call "XY Go.vi"("return immediately"=FALSE, "Speed"=w626, "XY In"=w625, "Gantry In"=w624) -> ("Gantry Out"=w623:refnum<k24>)  [unwired: 5 in, 2 out]
                      n145 = Delete From Array(array=w621, length=1, index=0) -> (array with subset deleted=w620:T3)  [unwired: 1 out]
                    }
                    frame True {
                      # "#7"
                      # "#2"
                      # "#1"
                      n146 = case shown="True" w647 {
                        tunnel: w655 -> [w666 w694]
                        tunnel: w654 -> [w663 w692]
                        tunnel: w653 -> [w662 w690]
                        tunnel: w652 -> [w660 w691]
                        tunnel: w651 -> [w659 w688]
                        tunnel: [w658 w689] -> w650
                        tunnel: [w657 w693] -> w649
                        tunnel: w648 -> [_ w687]
                        tunnel: w646 -> [_ w686]
                        tunnel: w645 -> [_ w685]
                        tunnel: w644 -> [_ w684]
                        tunnel: w643 -> [_ w683]
                        tunnel: w642 -> [_ w682]
                        tunnel: w641 -> [_ w681]
                        tunnel: w640 -> [_ w680]
                        tunnel: w639 -> [_ w679]
                        tunnel: w638 -> [_ w678]
                        tunnel: w637 -> [_ w677]
                        tunnel: w636 -> [_ w676]
                        tunnel: w635 -> [_ w675]
                        tunnel: w634 -> [_ w674]
                        tunnel: w633 -> [_ w673]
                        tunnel: w632 -> [_ w672]
                        tunnel: w631 -> [_ w671]
                        tunnel: w630 -> [_ w670]
                        tunnel: w629 -> [_ w669]
                        tunnel: w628 -> [_ w668]
                        tunnel: w627 -> [_ w667]
                        frame False {
                          w656 = FALSE ("return immediately")
                          n147 = call "XY Go.vi"("return immediately"=w656, "Speed"=w659, "XY In"=w663, "Gantry In"=w662) -> ("Gantry Out"=w661:refnum<k24>)  [unwired: 5 in, 2 out]
                          n148 = call "XY Go.vi"("return immediately"=w656, "Speed"=w659, "XY In"=w660, "Gantry In"=w661) -> ("Gantry Out"=w658:refnum<k24>)  [unwired: 5 in, 2 out]
                          n149 = Delete From Array(array=w666, length=2, index=0) -> (array with subset deleted=w657:T3)  [unwired: 1 out]
                        }
                        frame True {
                          # "#9"
                          # "#8"
                          # "#3"
                          # "#4"
                          # "#7"
                          n150 = case shown="True" w686 {
                            tunnel: w694 -> [w707 w728]
                            tunnel: [w704 w727] -> w693
                            tunnel: w692 -> [w703 w734]
                            tunnel: w691 -> [w702 w733]
                            tunnel: w690 -> [w701 w730]
                            tunnel: [w698 w729] -> w689
                            tunnel: w688 -> [w697 w731]
                            tunnel: w687 -> [w695 w732]
                            tunnel: w685 -> [_ w726]
                            tunnel: w684 -> [_ w725]
                            tunnel: w683 -> [_ w724]
                            tunnel: w682 -> [_ w723]
                            tunnel: w681 -> [_ w722]
                            tunnel: w680 -> [_ w721]
                            tunnel: w679 -> [_ w720]
                            tunnel: w678 -> [_ w719]
                            tunnel: w677 -> [_ w718]
                            tunnel: w676 -> [_ w717]
                            tunnel: w675 -> [_ w716]
                            tunnel: w674 -> [_ w715]
                            tunnel: w673 -> [_ w714]
                            tunnel: w672 -> [_ w713]
                            tunnel: w671 -> [_ w712]
                            tunnel: w670 -> [_ w711]
                            tunnel: w669 -> [_ w710]
                            tunnel: w668 -> [_ w709]
                            tunnel: w667 -> [_ w708]
                            frame False {
                              w696 = FALSE ("return immediately")
                              n151 = call "XY Go.vi"("return immediately"=w696, "Speed"=w697, "XY In"=w703, "Gantry In"=w701) -> ("Gantry Out"=w700:refnum<k24>)  [unwired: 5 in, 2 out]
                              n152 = call "XY Go.vi"("return immediately"=w696, "Speed"=w697, "XY In"=w702, "Gantry In"=w700) -> ("Gantry Out"=w699:refnum<k24>)  [unwired: 5 in, 2 out]
                              n153 = call "XY Go.vi"("return immediately"=w696, "Speed"=w697, "XY In"=w695, "Gantry In"=w699) -> ("Gantry Out"=w698:refnum<k24>)  [unwired: 5 in, 2 out]
                              n154 = Delete From Array(array=w707, length=3, index=0) -> (array with subset deleted=w704:T3)  [unwired: 1 out]
                            }
                            frame True {
                              # "#5"
                              # "#6"
                              n155 = case shown="True" w725 {
                                tunnel: w734 -> [w748 w772]
                                tunnel: w733 -> [w747 w771]
                                tunnel: w732 -> [w746 w770]
                                tunnel: w731 -> [w745 w768]
                                tunnel: w730 -> [w744 w767]
                                tunnel: [w740 w766] -> w729
                                tunnel: w728 -> [w737 w774]
                                tunnel: [w736 w773] -> w727
                                tunnel: w726 -> [w735 w769]
                                tunnel: w724 -> [_ w765]
                                tunnel: w723 -> [_ w764]
                                tunnel: w722 -> [_ w749]
                                tunnel: w721 -> [_ w763]
                                tunnel: w720 -> [_ w762]
                                tunnel: w719 -> [_ w761]
                                tunnel: w718 -> [_ w760]
                                tunnel: w717 -> [_ w759]
                                tunnel: w716 -> [_ w758]
                                tunnel: w715 -> [_ w757]
                                tunnel: w714 -> [_ w756]
                                tunnel: w713 -> [_ w755]
                                tunnel: w712 -> [_ w754]
                                tunnel: w711 -> [_ w753]
                                tunnel: w710 -> [_ w752]
                                tunnel: w709 -> [_ w751]
                                tunnel: w708 -> [_ w750]
                                frame False {
                                n156 = call "XY Go.vi"("Speed"=w745, "XY In"=w748, "Gantry In"=w744) -> ("Gantry Out"=w743:refnum<k24>)  [unwired: 6 in, 2 out]
                                n157 = call "XY Go.vi"("Speed"=w745, "XY In"=w747, "Gantry In"=w743) -> ("Gantry Out"=w742:refnum<k24>)  [unwired: 6 in, 2 out]
                                n158 = call "XY Go.vi"("Speed"=w745, "XY In"=w746, "Gantry In"=w742) -> ("Gantry Out"=w741:refnum<k24>)  [unwired: 6 in, 2 out]
                                n159 = call "XY Go.vi"("Speed"=w745, "XY In"=w735, "Gantry In"=w741) -> ("Gantry Out"=w740:refnum<k24>)  [unwired: 6 in, 2 out]
                                n160 = Delete From Array(array=w737, length=4, index=0) -> (array with subset deleted=w736:T3)  [unwired: 1 out]
                                }
                                frame True {
                                n161 = case shown="True" w764 {
                                tunnel: w774 -> [w790 w815]
                                tunnel: [w789 w814] -> w773
                                tunnel: w772 -> [w786 w813]
                                tunnel: w771 -> [w785 w812]
                                tunnel: w770 -> [w784 w810]
                                tunnel: w769 -> [w783 w809]
                                tunnel: w768 -> [w782 w808]
                                tunnel: w767 -> [w781 w807]
                                tunnel: [w776 w806] -> w766
                                tunnel: w765 -> [w775 w811]
                                tunnel: w749 -> [_ w805]
                                tunnel: w763 -> [_ w804]
                                tunnel: w762 -> [_ w803]
                                tunnel: w761 -> [_ w802]
                                tunnel: w760 -> [_ w801]
                                tunnel: w759 -> [_ w800]
                                tunnel: w758 -> [_ w799]
                                tunnel: w757 -> [_ w798]
                                tunnel: w756 -> [_ w797]
                                tunnel: w755 -> [_ w796]
                                tunnel: w754 -> [_ w795]
                                tunnel: w753 -> [_ w794]
                                tunnel: w752 -> [_ w793]
                                tunnel: w751 -> [_ w792]
                                tunnel: w750 -> [_ w791]
                                frame False {
                                n162 = call "XY Go.vi"("Speed"=w782, "XY In"=w786, "Gantry In"=w781) -> ("Gantry Out"=w780:refnum<k24>)  [unwired: 6 in, 2 out]
                                n163 = call "XY Go.vi"("Speed"=w782, "XY In"=w785, "Gantry In"=w780) -> ("Gantry Out"=w779:refnum<k24>)  [unwired: 6 in, 2 out]
                                n164 = call "XY Go.vi"("Speed"=w782, "XY In"=w784, "Gantry In"=w779) -> ("Gantry Out"=w778:refnum<k24>)  [unwired: 6 in, 2 out]
                                n165 = call "XY Go.vi"("Speed"=w782, "XY In"=w783, "Gantry In"=w778) -> ("Gantry Out"=w777:refnum<k24>)  [unwired: 6 in, 2 out]
                                n166 = call "XY Go.vi"("Speed"=w782, "XY In"=w775, "Gantry In"=w777) -> ("Gantry Out"=w776:refnum<k24>)  [unwired: 6 in, 2 out]
                                n167 = Delete From Array(array=w790, length=5, index=0) -> (array with subset deleted=w789:T3)  [unwired: 1 out]
                                }
                                frame True {
                                n168 = case shown="True" w804 {
                                tunnel: w815 -> [w831 w857]
                                tunnel: [w830 w856] -> w814
                                tunnel: w813 -> [w829 w855]
                                tunnel: w812 -> [w828 w854]
                                tunnel: w811 -> [w818 w853]
                                tunnel: w810 -> [w816 w852]
                                tunnel: w809 -> [w817 w850]
                                tunnel: w808 -> [w827 w849]
                                tunnel: w807 -> [w826 w848]
                                tunnel: [w820 w847] -> w806
                                tunnel: w805 -> [w819 w851]
                                tunnel: w803 -> [_ w846]
                                tunnel: w802 -> [_ w845]
                                tunnel: w801 -> [_ w844]
                                tunnel: w800 -> [_ w843]
                                tunnel: w799 -> [_ w842]
                                tunnel: w798 -> [_ w841]
                                tunnel: w797 -> [_ w840]
                                tunnel: w796 -> [_ w839]
                                tunnel: w795 -> [_ w838]
                                tunnel: w794 -> [_ w837]
                                tunnel: w793 -> [_ w836]
                                tunnel: w792 -> [_ w835]
                                tunnel: w791 -> [_ w834]
                                frame False {
                                n169 = call "XY Go.vi"("Speed"=w827, "XY In"=w829, "Gantry In"=w826) -> ("Gantry Out"=w825:refnum<k24>)  [unwired: 6 in, 2 out]
                                n170 = call "XY Go.vi"("Speed"=w827, "XY In"=w828, "Gantry In"=w825) -> ("Gantry Out"=w824:refnum<k24>)  [unwired: 6 in, 2 out]
                                n171 = call "XY Go.vi"("Speed"=w827, "XY In"=w816, "Gantry In"=w824) -> ("Gantry Out"=w823:refnum<k24>)  [unwired: 6 in, 2 out]
                                n172 = call "XY Go.vi"("Speed"=w827, "XY In"=w817, "Gantry In"=w823) -> ("Gantry Out"=w822:refnum<k24>)  [unwired: 6 in, 2 out]
                                n173 = call "XY Go.vi"("Speed"=w827, "XY In"=w818, "Gantry In"=w822) -> ("Gantry Out"=w821:refnum<k24>)  [unwired: 6 in, 2 out]
                                n174 = call "XY Go.vi"("Speed"=w827, "XY In"=w819, "Gantry In"=w821) -> ("Gantry Out"=w820:refnum<k24>)  [unwired: 6 in, 2 out]
                                n175 = Delete From Array(array=w831, length=6, index=0) -> (array with subset deleted=w830:T3)  [unwired: 1 out]
                                }
                                frame True {
                                n176 = case shown="True" w846 {
                                tunnel: w857 -> [w875 w890]
                                tunnel: [w874 w889] -> w856
                                tunnel: w855 -> [w873 w900]
                                tunnel: w854 -> [w872 w899]
                                tunnel: w853 -> [w858 w898]
                                tunnel: w852 -> [w860 w897]
                                tunnel: w851 -> [w859 w896]
                                tunnel: w850 -> [w861 w895]
                                tunnel: w849 -> [w871 w893]
                                tunnel: w848 -> [w870 w892]
                                tunnel: [w863 w891] -> w847
                                tunnel: w845 -> [w862 w894]
                                tunnel: w844 -> [_ w888]
                                tunnel: w843 -> [_ w887]
                                tunnel: w842 -> [_ w886]
                                tunnel: w841 -> [_ w885]
                                tunnel: w840 -> [_ w884]
                                tunnel: w839 -> [_ w883]
                                tunnel: w838 -> [_ w882]
                                tunnel: w837 -> [_ w881]
                                tunnel: w836 -> [_ w880]
                                tunnel: w835 -> [_ w879]
                                tunnel: w834 -> [_ w878]
                                frame False {
                                n177 = call "XY Go.vi"("Speed"=w871, "XY In"=w873, "Gantry In"=w870) -> ("Gantry Out"=w869:refnum<k24>)  [unwired: 6 in, 2 out]
                                n178 = call "XY Go.vi"("Speed"=w871, "XY In"=w872, "Gantry In"=w869) -> ("Gantry Out"=w868:refnum<k24>)  [unwired: 6 in, 2 out]
                                n179 = call "XY Go.vi"("Speed"=w871, "XY In"=w860, "Gantry In"=w868) -> ("Gantry Out"=w867:refnum<k24>)  [unwired: 6 in, 2 out]
                                n180 = call "XY Go.vi"("Speed"=w871, "XY In"=w861, "Gantry In"=w867) -> ("Gantry Out"=w866:refnum<k24>)  [unwired: 6 in, 2 out]
                                n181 = call "XY Go.vi"("Speed"=w871, "XY In"=w858, "Gantry In"=w866) -> ("Gantry Out"=w865:refnum<k24>)  [unwired: 6 in, 2 out]
                                n182 = call "XY Go.vi"("Speed"=w871, "XY In"=w859, "Gantry In"=w865) -> ("Gantry Out"=w864:refnum<k24>)  [unwired: 6 in, 2 out]
                                n183 = call "XY Go.vi"("Speed"=w871, "XY In"=w862, "Gantry In"=w864) -> ("Gantry Out"=w863:refnum<k24>)  [unwired: 6 in, 2 out]
                                n184 = Delete From Array(array=w875, length=7, index=0) -> (array with subset deleted=w874:T3)  [unwired: 1 out]
                                }
                                frame True {
                                n185 = case shown="True" w887 {
                                tunnel: w900 -> [w922 w942]
                                tunnel: w899 -> [w921 w941]
                                tunnel: w898 -> [w902 w940]
                                tunnel: w897 -> [w904 w939]
                                tunnel: w896 -> [w901 w938]
                                tunnel: w895 -> [w903 w937]
                                tunnel: w894 -> [w920 w936]
                                tunnel: w893 -> [w919 w934]
                                tunnel: w892 -> [w918 w933]
                                tunnel: [w910 w932] -> w891
                                tunnel: w890 -> [w907 w944]
                                tunnel: [w906 w943] -> w889
                                tunnel: w888 -> [w905 w935]
                                tunnel: w886 -> [_ w931]
                                tunnel: w885 -> [_ w930]
                                tunnel: w884 -> [_ w929]
                                tunnel: w883 -> [_ w928]
                                tunnel: w882 -> [_ w927]
                                tunnel: w881 -> [_ w926]
                                tunnel: w880 -> [_ w925]
                                tunnel: w879 -> [_ w924]
                                tunnel: w878 -> [_ w923]
                                frame False {
                                n186 = call "XY Go.vi"("Speed"=w919, "XY In"=w922, "Gantry In"=w918) -> ("Gantry Out"=w917:refnum<k24>)  [unwired: 6 in, 2 out]
                                n187 = call "XY Go.vi"("Speed"=w919, "XY In"=w921, "Gantry In"=w917) -> ("Gantry Out"=w916:refnum<k24>)  [unwired: 6 in, 2 out]
                                n188 = call "XY Go.vi"("Speed"=w919, "XY In"=w904, "Gantry In"=w916) -> ("Gantry Out"=w915:refnum<k24>)  [unwired: 6 in, 2 out]
                                n189 = call "XY Go.vi"("Speed"=w919, "XY In"=w903, "Gantry In"=w915) -> ("Gantry Out"=w914:refnum<k24>)  [unwired: 6 in, 2 out]
                                n190 = call "XY Go.vi"("Speed"=w919, "XY In"=w902, "Gantry In"=w914) -> ("Gantry Out"=w913:refnum<k24>)  [unwired: 6 in, 2 out]
                                n191 = call "XY Go.vi"("Speed"=w919, "XY In"=w901, "Gantry In"=w913) -> ("Gantry Out"=w912:refnum<k24>)  [unwired: 6 in, 2 out]
                                n192 = call "XY Go.vi"("Speed"=w919, "XY In"=w920, "Gantry In"=w912) -> ("Gantry Out"=w911:refnum<k24>)  [unwired: 6 in, 2 out]
                                n193 = call "XY Go.vi"("Speed"=w919, "XY In"=w905, "Gantry In"=w911) -> ("Gantry Out"=w910:refnum<k24>)  [unwired: 6 in, 2 out]
                                n194 = Delete From Array(array=w907, length=8, index=0) -> (array with subset deleted=w906:T3)  [unwired: 1 out]
                                }
                                frame True {
                                n195 = case shown="True" w930 {
                                tunnel: w944 -> [w968 w989]
                                tunnel: [w967 w988] -> w943
                                tunnel: w942 -> [w964 w987]
                                tunnel: w941 -> [w963 w986]
                                tunnel: w940 -> [w948 w985]
                                tunnel: w939 -> [w947 w984]
                                tunnel: w938 -> [w946 w983]
                                tunnel: w937 -> [w945 w982]
                                tunnel: w936 -> [w962 w981]
                                tunnel: w935 -> [w961 w980]
                                tunnel: w934 -> [w960 w978]
                                tunnel: w933 -> [w959 w977]
                                tunnel: [w950 w976] -> w932
                                tunnel: w931 -> [w949 w979]
                                tunnel: w929 -> [_ w975]
                                tunnel: w928 -> [_ w974]
                                tunnel: w927 -> [_ w973]
                                tunnel: w926 -> [_ w972]
                                tunnel: w925 -> [_ w971]
                                tunnel: w924 -> [_ w970]
                                tunnel: w923 -> [_ w969]
                                frame False {
                                n196 = call "XY Go.vi"("Speed"=w960, "XY In"=w964, "Gantry In"=w959) -> ("Gantry Out"=w958:refnum<k24>)  [unwired: 6 in, 2 out]
                                n197 = call "XY Go.vi"("Speed"=w960, "XY In"=w963, "Gantry In"=w958) -> ("Gantry Out"=w957:refnum<k24>)  [unwired: 6 in, 2 out]
                                n198 = call "XY Go.vi"("Speed"=w960, "XY In"=w947, "Gantry In"=w957) -> ("Gantry Out"=w956:refnum<k24>)  [unwired: 6 in, 2 out]
                                n199 = call "XY Go.vi"("Speed"=w960, "XY In"=w945, "Gantry In"=w956) -> ("Gantry Out"=w955:refnum<k24>)  [unwired: 6 in, 2 out]
                                n200 = call "XY Go.vi"("Speed"=w960, "XY In"=w948, "Gantry In"=w955) -> ("Gantry Out"=w954:refnum<k24>)  [unwired: 6 in, 2 out]
                                n201 = call "XY Go.vi"("Speed"=w960, "XY In"=w946, "Gantry In"=w954) -> ("Gantry Out"=w953:refnum<k24>)  [unwired: 6 in, 2 out]
                                n202 = call "XY Go.vi"("Speed"=w960, "XY In"=w962, "Gantry In"=w953) -> ("Gantry Out"=w952:refnum<k24>)  [unwired: 6 in, 2 out]
                                n203 = call "XY Go.vi"("Speed"=w960, "XY In"=w961, "Gantry In"=w952) -> ("Gantry Out"=w951:refnum<k24>)  [unwired: 6 in, 2 out]
                                n204 = call "XY Go.vi"("Speed"=w960, "XY In"=w949, "Gantry In"=w951) -> ("Gantry Out"=w950:refnum<k24>)  [unwired: 6 in, 2 out]
                                n205 = Delete From Array(array=w968, length=9, index=0) -> (array with subset deleted=w967:T3)  [unwired: 1 out]
                                }
                                frame True {
                                n206 = case shown="True" w974 {
                                tunnel: w989 -> [w1015 w1035]
                                tunnel: [w1012 w1034] -> w988
                                tunnel: w987 -> [w1011 w1031]
                                tunnel: w986 -> [w1010 w1030]
                                tunnel: w985 -> [w993 w1029]
                                tunnel: w984 -> [w992 w1028]
                                tunnel: w983 -> [w991 w1027]
                                tunnel: w982 -> [w990 w1026]
                                tunnel: w981 -> [w1009 w1025]
                                tunnel: w980 -> [w1008 w1024]
                                tunnel: w979 -> [w1007 w1023]
                                tunnel: w978 -> [w1006 w1021]
                                tunnel: w977 -> [w1005 w1033]
                                tunnel: [w995 w1032] -> w976
                                tunnel: w975 -> [w994 w1022]
                                tunnel: w973 -> [_ w1020]
                                tunnel: w972 -> [_ w1019]
                                tunnel: w971 -> [_ w1018]
                                tunnel: w970 -> [_ w1017]
                                tunnel: w969 -> [_ w1016]
                                frame False {
                                n207 = call "XY Go.vi"("Speed"=w1006, "XY In"=w1011, "Gantry In"=w1005) -> ("Gantry Out"=w1004:refnum<k24>)  [unwired: 6 in, 2 out]
                                n208 = Delete From Array(array=w1015, length=10, index=0) -> (array with subset deleted=w1012:T3)  [unwired: 1 out]
                                n209 = call "XY Go.vi"("Speed"=w1006, "XY In"=w1010, "Gantry In"=w1004) -> ("Gantry Out"=w1003:refnum<k24>)  [unwired: 6 in, 2 out]
                                n210 = call "XY Go.vi"("Speed"=w1006, "XY In"=w992, "Gantry In"=w1003) -> ("Gantry Out"=w1002:refnum<k24>)  [unwired: 6 in, 2 out]
                                n211 = call "XY Go.vi"("Speed"=w1006, "XY In"=w990, "Gantry In"=w1002) -> ("Gantry Out"=w1001:refnum<k24>)  [unwired: 6 in, 2 out]
                                n212 = call "XY Go.vi"("Speed"=w1006, "XY In"=w993, "Gantry In"=w1001) -> ("Gantry Out"=w1000:refnum<k24>)  [unwired: 6 in, 2 out]
                                n213 = call "XY Go.vi"("Speed"=w1006, "XY In"=w991, "Gantry In"=w1000) -> ("Gantry Out"=w999:refnum<k24>)  [unwired: 6 in, 2 out]
                                n214 = call "XY Go.vi"("Speed"=w1006, "XY In"=w1009, "Gantry In"=w999) -> ("Gantry Out"=w998:refnum<k24>)  [unwired: 6 in, 2 out]
                                n215 = call "XY Go.vi"("Speed"=w1006, "XY In"=w1008, "Gantry In"=w998) -> ("Gantry Out"=w997:refnum<k24>)  [unwired: 6 in, 2 out]
                                n216 = call "XY Go.vi"("Speed"=w1006, "XY In"=w1007, "Gantry In"=w997) -> ("Gantry Out"=w996:refnum<k24>)  [unwired: 6 in, 2 out]
                                n217 = call "XY Go.vi"("Speed"=w1006, "XY In"=w994, "Gantry In"=w996) -> ("Gantry Out"=w995:refnum<k24>)  [unwired: 6 in, 2 out]
                                }
                                frame True {
                                n218 = case shown="True" w1019 {
                                tunnel: w1035 -> [w1063 w1082]
                                tunnel: [w1060 w1081] -> w1034
                                tunnel: w1033 -> [w1059 w1069]
                                tunnel: [w1048 w1068] -> w1032
                                tunnel: w1031 -> [w1047 w1080]
                                tunnel: w1030 -> [w1046 w1079]
                                tunnel: w1029 -> [w1040 w1078]
                                tunnel: w1028 -> [w1038 w1077]
                                tunnel: w1027 -> [w1039 w1076]
                                tunnel: w1026 -> [w1041 w1075]
                                tunnel: w1025 -> [w1045 w1074]
                                tunnel: w1024 -> [w1044 w1073]
                                tunnel: w1023 -> [w1036 w1072]
                                tunnel: w1022 -> [w1037 w1071]
                                tunnel: w1021 -> [w1043 w1064]
                                tunnel: w1020 -> [w1042 w1070]
                                tunnel: w1018 -> [_ w1067]
                                tunnel: w1017 -> [_ w1066]
                                tunnel: w1016 -> [_ w1065]
                                frame False {
                                n219 = call "XY Go.vi"("Speed"=w1043, "XY In"=w1047, "Gantry In"=w1059) -> ("Gantry Out"=w1058:refnum<k24>)  [unwired: 6 in, 2 out]
                                n220 = Delete From Array(array=w1063, length=11, index=0) -> (array with subset deleted=w1060:T3)  [unwired: 1 out]
                                n221 = call "XY Go.vi"("Speed"=w1043, "XY In"=w1046, "Gantry In"=w1058) -> ("Gantry Out"=w1057:refnum<k24>)  [unwired: 6 in, 2 out]
                                n222 = call "XY Go.vi"("Speed"=w1043, "XY In"=w1038, "Gantry In"=w1057) -> ("Gantry Out"=w1056:refnum<k24>)  [unwired: 6 in, 2 out]
                                n223 = call "XY Go.vi"("Speed"=w1043, "XY In"=w1041, "Gantry In"=w1056) -> ("Gantry Out"=w1055:refnum<k24>)  [unwired: 6 in, 2 out]
                                n224 = call "XY Go.vi"("Speed"=w1043, "XY In"=w1040, "Gantry In"=w1055) -> ("Gantry Out"=w1054:refnum<k24>)  [unwired: 6 in, 2 out]
                                n225 = call "XY Go.vi"("Speed"=w1043, "XY In"=w1039, "Gantry In"=w1054) -> ("Gantry Out"=w1053:refnum<k24>)  [unwired: 6 in, 2 out]
                                n226 = call "XY Go.vi"("Speed"=w1043, "XY In"=w1045, "Gantry In"=w1053) -> ("Gantry Out"=w1052:refnum<k24>)  [unwired: 6 in, 2 out]
                                n227 = call "XY Go.vi"("Speed"=w1043, "XY In"=w1044, "Gantry In"=w1052) -> ("Gantry Out"=w1051:refnum<k24>)  [unwired: 6 in, 2 out]
                                n228 = call "XY Go.vi"("Speed"=w1043, "XY In"=w1036, "Gantry In"=w1051) -> ("Gantry Out"=w1050:refnum<k24>)  [unwired: 6 in, 2 out]
                                n229 = call "XY Go.vi"("Speed"=w1043, "XY In"=w1037, "Gantry In"=w1050) -> ("Gantry Out"=w1049:refnum<k24>)  [unwired: 6 in, 2 out]
                                n230 = call "XY Go.vi"("Speed"=w1043, "XY In"=w1042, "Gantry In"=w1049) -> ("Gantry Out"=w1048:refnum<k24>)  [unwired: 6 in, 2 out]
                                }
                                frame True {
                                n231 = case shown="True" w1066 {
                                tunnel: w1082 -> [w1111 w1144]
                                tunnel: [w1110 w1143] -> w1081
                                tunnel: w1080 -> [w1109 w1142]
                                tunnel: w1079 -> [w1108 w1141]
                                tunnel: w1078 -> [w1085 w1116]
                                tunnel: w1077 -> [w1083 w1114]
                                tunnel: w1076 -> [w1084 w1117]
                                tunnel: w1075 -> [w1086 w1115]
                                tunnel: w1074 -> [w1107 w1140]
                                tunnel: w1073 -> [w1106 w1139]
                                tunnel: w1072 -> [w1105 w1138]
                                tunnel: w1071 -> [w1104 w1137]
                                tunnel: w1070 -> [w1103 w1136]
                                tunnel: w1069 -> [w1102 w1133]
                                tunnel: [w1090 w1120] -> w1068
                                tunnel: w1067 -> [w1089 w1135]
                                tunnel: w1065 -> [_ w1134]
                                tunnel: w1064 -> [w1087 w1119]
                                frame False {
                                w1088 = FALSE
                                n232 = call "XY Go.vi"("return immediately"=w1088, "Speed"=w1087, "XY In"=w1109, "Gantry In"=w1102) -> ("Gantry Out"=w1101:refnum<k24>)  [unwired: 5 in, 2 out]
                                n233 = Delete From Array(array=w1111, length=12, index=0) -> (array with subset deleted=w1110:T3)  [unwired: 1 out]
                                n234 = call "XY Go.vi"("return immediately"=w1088, "Speed"=w1087, "XY In"=w1108, "Gantry In"=w1101) -> ("Gantry Out"=w1100:refnum<k24>)  [unwired: 5 in, 2 out]
                                n235 = call "XY Go.vi"("return immediately"=w1088, "Speed"=w1087, "XY In"=w1083, "Gantry In"=w1100) -> ("Gantry Out"=w1099:refnum<k24>)  [unwired: 5 in, 2 out]
                                n236 = call "XY Go.vi"("return immediately"=w1088, "Speed"=w1087, "XY In"=w1086, "Gantry In"=w1099) -> ("Gantry Out"=w1098:refnum<k24>)  [unwired: 5 in, 2 out]
                                n237 = call "XY Go.vi"("return immediately"=w1088, "Speed"=w1087, "XY In"=w1085, "Gantry In"=w1098) -> ("Gantry Out"=w1097:refnum<k24>)  [unwired: 5 in, 2 out]
                                n238 = call "XY Go.vi"("return immediately"=w1088, "Speed"=w1087, "XY In"=w1084, "Gantry In"=w1097) -> ("Gantry Out"=w1096:refnum<k24>)  [unwired: 5 in, 2 out]
                                n239 = call "XY Go.vi"("return immediately"=w1088, "Speed"=w1087, "XY In"=w1107, "Gantry In"=w1096) -> ("Gantry Out"=w1095:refnum<k24>)  [unwired: 5 in, 2 out]
                                n240 = call "XY Go.vi"("return immediately"=w1088, "Speed"=w1087, "XY In"=w1106, "Gantry In"=w1095) -> ("Gantry Out"=w1094:refnum<k24>)  [unwired: 5 in, 2 out]
                                n241 = call "XY Go.vi"("return immediately"=w1088, "Speed"=w1087, "XY In"=w1105, "Gantry In"=w1094) -> ("Gantry Out"=w1093:refnum<k24>)  [unwired: 5 in, 2 out]
                                n242 = call "XY Go.vi"("return immediately"=w1088, "Speed"=w1087, "XY In"=w1104, "Gantry In"=w1093) -> ("Gantry Out"=w1092:refnum<k24>)  [unwired: 5 in, 2 out]
                                n243 = call "XY Go.vi"("return immediately"=w1088, "Speed"=w1087, "XY In"=w1103, "Gantry In"=w1092) -> ("Gantry Out"=w1091:refnum<k24>)  [unwired: 5 in, 2 out]
                                n244 = call "XY Go.vi"("return immediately"=w1088, "Speed"=w1087, "XY In"=w1089, "Gantry In"=w1091) -> ("Gantry Out"=w1090:refnum<k24>)  [unwired: 5 in, 2 out]
                                }
                                frame True {
                                w1118 = FALSE
                                n245 = Delete From Array(array=w1144, length=13, index=0) -> (array with subset deleted=w1143:T3)  [unwired: 1 out]
                                n246 = call "XY Go.vi"("return immediately"=w1118, "Speed"=w1119, "XY In"=w1142, "Gantry In"=w1133) -> ("Gantry Out"=w1132:refnum<k24>)  [unwired: 5 in, 2 out]
                                n247 = call "XY Go.vi"("return immediately"=w1118, "Speed"=w1119, "XY In"=w1141, "Gantry In"=w1132) -> ("Gantry Out"=w1131:refnum<k24>)  [unwired: 5 in, 2 out]
                                n248 = call "XY Go.vi"("return immediately"=w1118, "Speed"=w1119, "XY In"=w1114, "Gantry In"=w1131) -> ("Gantry Out"=w1130:refnum<k24>)  [unwired: 5 in, 2 out]
                                n249 = call "XY Go.vi"("return immediately"=w1118, "Speed"=w1119, "XY In"=w1115, "Gantry In"=w1130) -> ("Gantry Out"=w1129:refnum<k24>)  [unwired: 5 in, 2 out]
                                n250 = call "XY Go.vi"("return immediately"=w1118, "Speed"=w1119, "XY In"=w1116, "Gantry In"=w1129) -> ("Gantry Out"=w1128:refnum<k24>)  [unwired: 5 in, 2 out]
                                n251 = call "XY Go.vi"("return immediately"=w1118, "Speed"=w1119, "XY In"=w1117, "Gantry In"=w1128) -> ("Gantry Out"=w1127:refnum<k24>)  [unwired: 5 in, 2 out]
                                n252 = call "XY Go.vi"("return immediately"=w1118, "Speed"=w1119, "XY In"=w1140, "Gantry In"=w1127) -> ("Gantry Out"=w1126:refnum<k24>)  [unwired: 5 in, 2 out]
                                n253 = call "XY Go.vi"("return immediately"=w1118, "Speed"=w1119, "XY In"=w1139, "Gantry In"=w1126) -> ("Gantry Out"=w1125:refnum<k24>)  [unwired: 5 in, 2 out]
                                n254 = call "XY Go.vi"("return immediately"=w1118, "Speed"=w1119, "XY In"=w1138, "Gantry In"=w1125) -> ("Gantry Out"=w1124:refnum<k24>)  [unwired: 5 in, 2 out]
                                n255 = call "XY Go.vi"("return immediately"=w1118, "Speed"=w1119, "XY In"=w1137, "Gantry In"=w1124) -> ("Gantry Out"=w1123:refnum<k24>)  [unwired: 5 in, 2 out]
                                n256 = call "XY Go.vi"("return immediately"=w1118, "Speed"=w1119, "XY In"=w1136, "Gantry In"=w1123) -> ("Gantry Out"=w1122:refnum<k24>)  [unwired: 5 in, 2 out]
                                n257 = call "XY Go.vi"("return immediately"=w1118, "Speed"=w1119, "XY In"=w1135, "Gantry In"=w1122) -> ("Gantry Out"=w1121:refnum<k24>)  [unwired: 5 in, 2 out]
                                n258 = call "XY Go.vi"("return immediately"=w1118, "Speed"=w1119, "XY In"=w1134, "Gantry In"=w1121) -> ("Gantry Out"=w1120:refnum<k24>)  [unwired: 5 in, 2 out]
                                }
                                }
                                }
                                }
                                }
                                }
                                }
                                }
                                }
                                }
                                }
                                }
                                }
                                }
                                }
                                }
                                }
                              }
                            }
                          }
                        }
                      }
                    }
                  }
                  n259 = flat-sequence {
                    tunnel: [w1147] -> w616
                    tunnel: [w1151] -> w613
                    tunnel: [w1150] -> w610
                    tunnel: w615 -> [w1152]
                    tunnel: w612 -> [w1151]
                    tunnel: w609 -> [w1150]
                    tunnel: w604 -> [w1148]
                    tunnel: w577 -> [w1147]
                    tunnel: [w1156] -> w617
                    tunnel: w616 -> [w1155]
                    tunnel: [w1154] -> w614
                    tunnel: w613 -> [w1154]
                    tunnel: [w1153] -> w611
                    tunnel: w610 -> [w1153]
                    frame #0 {
                      n260 = Subtract(x=w1152, y=w1148) -> (x-y=w1149:i32)
                      n261 = Wait (ms)(milliseconds to wait=w1149) -> ()  [unwired: 1 out]
                    }
                    frame #1 {
                      n262 = call "Dispense.vi"("Dispenser In"=w1155) -> ("Dispenser Out"=w1156:refnum<visa-resource-name>)  [unwired: 9 in, 1 out]
                    }
                  }
                }
                frame #3 {
                  n263 = Negate(x=w1161) -> (-x=w1160:dbl)
                  n264 = call "Z Go.vi"("Increment"=TRUE, "Return Immediately"=FALSE, "Speed In"=w1159, "Position In"=w1160, "Gantry In"=w1162) -> ("Gantry Out"=w1164:refnum<k24>)  [unwired: 3 in, 3 out]
                }
              }
            }
            frame "Arc" {
              n265 = Index Array(array=w1194) -> (element #1=w1173:dbl[], element #2=w1188:dbl[])  [unwired: 4 in]
              n266 = flat-sequence {
                tunnel: [w1212] -> w1204
                tunnel: w1196 -> [w1211]
                tunnel: w1195 -> [w1210]
                tunnel: w1173 -> [w1209]
                tunnel: w1193 -> [w1208]
                tunnel: [w1207] -> w1180
                tunnel: w1179 -> [w1206]
                tunnel: w1178 -> [w1205]
                tunnel: w1204 -> [w1238]
                tunnel: [w1239] -> w1203
                tunnel: [w1235] -> w1202
                tunnel: [w1232] -> w1201
                tunnel: [w1229] -> w1200
                tunnel: w1192 -> [w1228]
                tunnel: w1191 -> [w1227]
                tunnel: w1190 -> [w1226]
                tunnel: w1189 -> [w1225]
                tunnel: w1180 -> [w1224]
                tunnel: w1203 -> [w1282]
                tunnel: [w1283] -> w1199
                tunnel: w1202 -> [w1273]
                tunnel: w1201 -> [w1286]
                tunnel: [w1286] -> w1198
                tunnel: w1200 -> [w1285]
                tunnel: [w1285] -> w1197
                tunnel: w1188 -> [w1276]
                tunnel: w1187 -> [w1275]
                tunnel: w1186 -> [w1277]
                tunnel: w1185 -> [w1279]
                tunnel: w1184 -> [w1284]
                tunnel: [w1274] -> w1181
                tunnel: w1177 -> [w1280]
                tunnel: w1176 -> [w1272]
                tunnel: w1175 -> [w1271]
                tunnel: w1174 -> [w1270]
                tunnel: w1173 -> [w1269]
                tunnel: w1172 -> [w1268]
                tunnel: w1171 -> [w1267]
                tunnel: w1170 -> [w1266]
                tunnel: w1169 -> [w1265]
                tunnel: w1168 -> [w1264]
                tunnel: w1167 -> [w1263]
                tunnel: [w1262] -> w1166
                tunnel: w1165 -> [w1261]
                tunnel: [w1395] -> w1183
                tunnel: w1199 -> [w1394]
                tunnel: [w1394] -> w1182
                tunnel: w1198 -> [w1392]
                tunnel: w1197 -> [w1390]
                tunnel: w1181 -> [w1393]
                frame #0 {
                  n267 = call "Pressure.vi"("Pressure"=w1205, "VISA resource name"=w1206) -> ("VISA resource name out"=w1207:refnum<visa-resource-name>)  [unwired: 8 in, 1 out]
                  n268 = case shown="True" w1211 {
                    tunnel: [w1217 w1221] -> w1212
                    tunnel: w1210 -> [w1216 w1220]
                    tunnel: w1209 -> [w1215 w1219]
                    tunnel: w1208 -> [w1214 _]
                    frame False {
                      n269 = call "XY Go.vi"("return immediately"=FALSE, "Speed"=w1214, "XY In"=w1215, "Gantry In"=w1216) -> ("Gantry Out"=w1217:refnum<k24>)  [unwired: 5 in, 2 out]
                    }
                    frame True {
                      n270 = call "ClearXYZTheta Go.vi"("Speed"=300.0, "XYZTheta In"=w1219, "Gantry In"=w1220) -> ("Gantry Out"=w1221:refnum<k24>)  [unwired: 6 in, 2 out]
                    }
                  }
                }
                frame #1 {
                  n271 = flat-sequence {
                    tunnel: w1238 -> [w1248]
                    tunnel: [w1246] -> w1237
                    tunnel: [w1245] -> w1234
                    tunnel: [w1244] -> w1233
                    tunnel: w1226 -> [w1243]
                    tunnel: w1225 -> [w1242]
                    tunnel: w1224 -> [w1240]
                    tunnel: [w1240] -> w1223
                    tunnel: w1237 -> [w1255]
                    tunnel: [w1255] -> w1236
                    tunnel: w1234 -> [w1254]
                    tunnel: w1233 -> [w1253]
                    tunnel: [w1254] -> w1231
                    tunnel: [w1253] -> w1230
                    tunnel: w1228 -> [w1252]
                    tunnel: w1227 -> [w1251]
                    tunnel: w1223 -> [w1250]
                    tunnel: [w1250] -> w1222
                    tunnel: [w1260] -> w1239
                    tunnel: w1236 -> [w1259]
                    tunnel: [w1259] -> w1235
                    tunnel: [w1258] -> w1232
                    tunnel: w1231 -> [w1258]
                    tunnel: w1230 -> [w1257]
                    tunnel: [w1257] -> _
                    tunnel: [w1257] -> w1229
                    tunnel: w1222 -> [w1256]
                    frame #0 {
                      n272 = call "Z Go.vi"("Increment"=TRUE, "Return Immediately"=TRUE, "Speed In"=w1242, "Position In"=w1243, "Gantry In"=w1248) -> ("Speed Out"=w1244:dbl, "Position Out"=w1245:dbl, "Gantry Out"=w1246:refnum<k24>)  [unwired: 3 in, 1 out]
                    }
                    frame #1 {
                      n273 = Subtract(x=w1252, y=w1251) -> (x-y=w1249:i32)
                      n274 = Wait (ms)(milliseconds to wait=w1249) -> ()  [unwired: 1 out]
                    }
                    frame #2 {
                      n275 = call "Dispense.vi"("Dispenser In"=w1256) -> ("Dispenser Out"=w1260:refnum<visa-resource-name>)  [unwired: 9 in, 1 out]
                    }
                  }
                }
                frame #2 {
                  n276 = flat-sequence {
                    tunnel: [w1383] -> w1281
                    tunnel: w1284 -> [w1385]
                    tunnel: w1282 -> [w1383]
                    tunnel: w1280 -> [w1382]
                    tunnel: [w1387] -> w1283
                    tunnel: w1281 -> [w1386]
                    frame #0 {
                      n277 = Subtract(x=w1385, y=w1382) -> (x-y=w1384:i32)
                      n278 = Wait (ms)(milliseconds to wait=w1384) -> ()  [unwired: 1 out]
                    }
                    frame #1 {
                      n279 = call "Dispense.vi"("Dispenser In"=w1386) -> ("Dispenser Out"=w1387:refnum<visa-resource-name>)  [unwired: 9 in, 1 out]
                    }
                  }
                  n280 = case shown="True" w1266 {
                    tunnel: w1279 -> [w1297 w1312]
                    tunnel: FALSE ("return immediately") -> [w1296 _]
                    tunnel: w1277 -> [w1295 w1311]
                    tunnel: w1276 -> [w1294 w1313]
                    tunnel: w1275 -> [w1293 w1314]
                    tunnel: [w1292 w1301] -> w1274
                    tunnel: w1273 -> [w1291 w1302]
                    tunnel: w1272 -> [_ w1310]
                    tunnel: w1271 -> [_ w1309]
                    tunnel: w1270 -> [_ w1308]
                    tunnel: w1269 -> [_ w1307]
                    tunnel: w1268 -> [_ w1306]
                    tunnel: w1267 -> [_ w1305]
                    tunnel: w1265 -> [_ w1304]
                    tunnel: w1264 -> [_ w1303]
                    tunnel: w1263 -> [w1290 w1300]
                    tunnel: [w1287 w1299] -> w1262
                    tunnel: w1261 -> [_ w1298]
                    frame False {
                      n281 = call "Circular.vi"("Direction"=w1297, "return immediately"=w1296, "Speed"=w1295, "XY End"=w1294, "XY Center"=w1293, "Gantry In"=w1291) -> ("Gantry Out"=w1292:refnum<k24>)  [unwired: 4 in, 1 out]
                      n282 = Delete From Array(array=w1290, length=1, index=0) -> (array with subset deleted=w1287:T3)  [unwired: 1 out]
                    }
                    frame True {
                      n283 = case shown="True" w1304 {
                        tunnel: w1314 -> [w1328 w1342]
                        tunnel: w1313 -> [w1327 w1341]
                        tunnel: w1312 -> [w1326 w1332]
                        tunnel: w1311 -> [w1325 w1333]
                        tunnel: w1310 -> [w1323 w1343]
                        tunnel: w1309 -> [w1322 w1344]
                        tunnel: w1308 -> [_ w1340]
                        tunnel: w1307 -> [_ w1339]
                        tunnel: w1306 -> [_ w1338]
                        tunnel: w1305 -> [_ w1337]
                        tunnel: w1303 -> [_ w1336]
                        tunnel: w1302 -> [w1321 w1335]
                        tunnel: [w1319 w1334] -> w1301
                        tunnel: w1300 -> [w1318 w1331]
                        tunnel: [w1317 w1330] -> w1299
                        tunnel: w1298 -> [_ w1329]
                        frame False {
                          w1324 = FALSE
                          n284 = call "Circular.vi"("Direction"=w1326, "return immediately"=w1324, "Speed"=w1325, "XY End"=w1327, "XY Center"=w1328, "Gantry In"=w1321) -> ("Gantry Out"=w1320:refnum<k24>)  [unwired: 4 in, 1 out]
                          n285 = call "Circular.vi"("Direction"=w1326, "return immediately"=w1324, "Speed"=w1325, "XY End"=w1323, "XY Center"=w1322, "Gantry In"=w1320) -> ("Gantry Out"=w1319:refnum<k24>)  [unwired: 4 in, 1 out]
                          n286 = Delete From Array(array=w1318, length=2, index=0) -> (array with subset deleted=w1317:T3)  [unwired: 1 out]
                        }
                        frame True {
                          n287 = case shown="True" w1336 {
                            tunnel: w1344 -> [w1360 w1381]
                            tunnel: w1343 -> [w1357 w1380]
                            tunnel: w1342 -> [w1359 w1379]
                            tunnel: w1341 -> [w1358 w1378]
                            tunnel: w1340 -> [w1361 w1377]
                            tunnel: w1339 -> [_ _]
                            tunnel: w1338 -> [_ w1376]
                            tunnel: w1337 -> [_ w1375]
                            tunnel: w1335 -> [w1356 w1374]
                            tunnel: [w1353 w1370] -> w1334
                            tunnel: w1333 -> [w1352 w1369]
                            tunnel: w1332 -> [w1351 w1368]
                            tunnel: w1331 -> [w1349 w1366]
                            tunnel: [w1348 w1365] -> w1330
                            tunnel: w1329 -> [w1345 w1362]
                            frame False {
                              w1350 = FALSE
                              n288 = call "Circular.vi"("Direction"=w1351, "return immediately"=w1350, "Speed"=w1352, "XY End"=w1358, "XY Center"=w1359, "Gantry In"=w1356) -> ("Gantry Out"=w1355:refnum<k24>)  [unwired: 4 in, 1 out]
                              n289 = call "Circular.vi"("Direction"=w1351, "return immediately"=w1350, "Speed"=w1352, "XY End"=w1357, "XY Center"=w1360, "Gantry In"=w1355) -> ("Gantry Out"=w1354:refnum<k24>)  [unwired: 4 in, 1 out]
                              n290 = call "Circular.vi"("Direction"=w1351, "return immediately"=w1350, "Speed"=w1352, "XY End"=w1345, "XY Center"=w1361, "Gantry In"=w1354) -> ("Gantry Out"=w1353:refnum<k24>)  [unwired: 4 in, 1 out]
                              n291 = Delete From Array(array=w1349, length=3, index=0) -> (array with subset deleted=w1348:T3)  [unwired: 1 out]
                            }
                            frame True {
                              w1367 = FALSE
                              n292 = Delete From Array(array=w1366, length=4, index=0) -> (array with subset deleted=w1365:T3)  [unwired: 1 out]
                              n293 = call "Circular.vi"("Direction"=w1368, "return immediately"=w1367, "Speed"=w1369, "XY End"=w1378, "XY Center"=w1379, "Gantry In"=w1374) -> ("Gantry Out"=w1373:refnum<k24>)  [unwired: 4 in, 1 out]
                              n294 = call "Circular.vi"("Direction"=w1368, "return immediately"=w1367, "Speed"=w1369, "XY End"=w1380, "XY Center"=w1381, "Gantry In"=w1373) -> ("Gantry Out"=w1372:refnum<k24>)  [unwired: 4 in, 1 out]
                              n295 = call "Circular.vi"("Direction"=w1368, "return immediately"=w1367, "Speed"=w1369, "XY End"=w1362, "XY Center"=w1377, "Gantry In"=w1372) -> ("Gantry Out"=w1371:refnum<k24>)  [unwired: 4 in, 1 out]
                              n296 = call "Circular.vi"("Direction"=w1368, "return immediately"=w1367, "Speed"=w1369, "XY End"=w1375, "XY Center"=w1376, "Gantry In"=w1371) -> ("Gantry Out"=w1370:refnum<k24>)  [unwired: 4 in, 1 out]
                            }
                          }
                        }
                      }
                    }
                  }
                }
                frame #3 {
                  n297 = Negate(x=w1392) -> (-x=w1391:dbl)
                  n298 = call "Z Go.vi"("Increment"=TRUE, "Return Immediately"=FALSE, "Speed In"=w1390, "Position In"=w1391, "Gantry In"=w1393) -> ("Gantry Out"=w1395:refnum<k24>)  [unwired: 3 in, 3 out]
                }
              }
            }
          }
          n299 = Array Size(array=w116) -> (size(s)=w117:i32)
          n300 = Equal To 0?(x=w117) -> (x = 0?=w118:bool)
        }
        n301 = in-place-cluster #1("Gantry"=w22, "Dispenser"=w18) -> (w9:T2)
      }
    }
    frame Error {
    }
  }
  "error out" <- w2
  "Sensor Dispense out" <- w5
  "Control Out" <- w3
